vi "Main.vi"() -> ()   [LabVIEW 2015]
uses:
  XYZStage/XYZStage Configuration.ctl
  Camera/Acquisition Settings.ctl
  Automation/ZO Settings.ctl
  Automation/Zstack Settings.ctl
  AOD/AOD Configuration.ctl
  controls/UI Data.ctl
  controls/UI State.ctl
  Settings/Settings.ctl
  Camera/Camera Configuration.ctl
  Logging/Logging Configuration.ctl
  DM/DM Configuration.ctl
  Automation/Automation Configuration.ctl
  V7001/V7001 Configuration.ctl
  <vilib>/vision/Image Controls.llb/IMAQ Image.ctl
  Camera/Camera State.ctl
  Camera/Camera Loop State.ctl
  <vilib>/Utility/miscctls.llb/LVMinMaxIncTypeDef.ctl
  Camera/Live View State.ctl
  DM/DM State.ctl
  DM/DM Loop State.ctl
  V7001/V7001 State.ctl
  V7001/V7001 Loop State.ctl
  AOD/AOD State.ctl
  AOD/AOD Loop State.ctl
  XYZStage/XYZStage State.ctl
  XYZStage/XYZStage Loop State.ctl
  <vilib>/Utility/error.llb/Error Cluster From Error Code.vi
  <vilib>/ErrorRing/Error Ring.xnode
  support/User Event - Stop/Copy of User Event - Stop.lvlib
  support/Message Queue/Message Queue.lvlib
  Camera/Camera.lvlib
  Settings/Settings.lvlib
  Logging/Logging.lvlib
  XYZStage/XYZStage.lvlib
  DM/DM.lvlib
  Automation/Automation.lvlib
  <vilib>/vision/NI_Vision_Development_Module.lvlib
  V7001/V7001.lvlib
  AOD/AOD.lvlib
panel:
  out "Camera Status":bool
  in  "Connect Camera":bool
  in  "X,Y":dbl[](array[slide])=[0.0, 0.0, 0.0, 0.0, 0.0, -0.06565656565656566, 0.0, 0.0, 0.043434343434343436, 0.0, 0.0, 0.0, 0.0, 0.0, 0.0] min=-1.0 max=1.0 scale=-1.0..1.0
  out "AOD Status":string="Disconnected"
  in  "AOD Configuration":T1={"Physical Channel"="Dev1/ao0:1", "Maximum Value"=10.0, "Minimum Value"=1.0, "Update Rate"=192000.0} {"Update Rate" format="%0.2f"; "Minimum Value" format="%0.2f"; "Maximum Value" format="%0.2f"}
  out "AOD Status":bool
  in  "Connect AOD":bool
  in  "Frame":u16(ring)=2 items=["All Off", "All On", "Checkerboard 1", "Random"]
  in  "Test Frame":bool
  out "V7001 Status":string="Disconnected"
  out "V7001 Status":bool
  in  "Connect DMD":bool
  out "XYZ notification":dbl[](array[numeric])
  in  "Move To":bool
  in  "Position in Microns 2":dbl[](array[numeric])
  out "Position in Microns":dbl[](array[numeric])
  in  "Tab Control 2":enum32{"Zernike", "Zstack"}(tab)=enum."Zstack"
  in  "Project and record":bool
  in  "ZO Settings":T2={"Acquisition Settings"={"Save?"=TRUE, "DCIMG Path"=path "E:/test2", "Filename"="beads", "Total Frames"=0, "Sender"=enum."UI"}, "Shift Amplitude"=0.1, "Initial Zernike Vector"=[0.0, 0.0, 0.0, 0.0, 0.0, 0.0, 0.0, 0.0, 0.0, 0.0, 0.0, 0.0, 0.0, 0.0, 0.0]}
  in  "Take Z Stack":bool
  in  "Stop at Current Pos":bool
  in  "Start at Current Pos":bool
  in  "Zstack Settings":T4={"Acquisition Settings"={"Save?"=TRUE, "DCIMG Path"=path "E:/test3", "Filename"="zstacktest1", "Total Frames"=10, "Sender"=enum."UI"}, "XYZ start"=[100.0, 100.0, 100.0], "XYZ end"=[100.0, 100.0, 8282.6875]}
  in  "Stage Stop":bool
  in  "step.size.xy":u16(ring)=6 items=["  1"=1, "  2"=2, "  5"=5, " 10"=10, " 20"=20, " 50"=50, "100"=100]
  in  "Y UP":bool
  in  "X LEFT":bool
  in  "Y DOWN":bool
  in  "X RIGHT":bool
  in  "step.size.z":u16(ring)=6 items=["  1"=1, "  2"=2, "  5"=5, " 10"=10, " 20"=20, " 50"=50, "100"=100]
  in  "Z UP":bool
  in  "Z DOWN":bool
  out "(Basic Histogram)":T5(graph)
  out "Automation Status":string
  in  "Tab Control":enum32{"Manual Trigger", "Live Mode"}(tab)
  in  "Exposure":dbl
  in  "Acquisition Settings":T3={"Save?"=FALSE, "DCIMG Path"=path "E:/test2", "Filename"="test", "Total Frames"=15, "Sender"=enum."UI"}
  in  "Acquire frames":bool
  in  "snap":bool
  out "Acquired Frames":dbl
  in  "Cancel Sequence":bool
  out "Camera Status 3":string
  in  "Go Live":bool
  out "Display":T6(plugin-control)
  in  "Connect DM":bool
  out "Intensity Graph":dbl[][](graph)=[[0.5, 0.5, 0.5, 0.5159398573354096, 0.5288164557874044, 0.535167056900559, 0.5377202162789856, 0.53921067600134, 0.5423702911567251, 0.5, 0.5, 0.5], [0.5, 0.5, 0.4975915358440764, 0.5151805163221181, 0.5235020295826256, 0.5252975455042929, 0.5232956196912321, 0.5202309942220992, 0.5188355241859969, 0.5218457302341335, 0.5, 0.5], [0.5, 0.47468889730160246, 0.5006284404962225, 0.5145729816339067, 0.5192500555540568, 0.5174011321353665, 0.5117547669819483, 0.505045702172458, 0.5000057927959983, 0.49937155950377754, 0.5058738366201876, 0.5], [0.44177297969755197, 0.4797001888362955, 0.5029062478643276, 0.514117304835424, 0.5160608945889862, 0.511478487003708, 0.5030986376837019, 0.4936560887076236, 0.48588269516457605, 0.48251497770576735, 0.48628377065558953, 0.49991687181031336], [0.44693499496071193, 0.4830402937519164, 0.5044244424324095, 0.5138135890559667, 0.5139352684619899, 0.5075309505291726, 0.49732919086162747, 0.4860647315380101, 0.4764694276474235, 0.4712797998410757, 0.4732266824433588, 0.4850378732505436], [0.4495168789955624, 0.4847109132903577, 0.5051837974744415, 0.5136616796015896, 0.5128720945112036, 0.5055565120819772, 0.4944434879180228, 0.4822677640979963, 0.4717611957110005, 0.46566030340824355, 0.46669592151411743, 0.47759584782489306], [0.4495168789955624, 0.4847109132903577, 0.5051837974744415, 0.5136616796015896, 0.5128720945112036, 0.5055565120819772, 0.4944434879180228, 0.4822677640979963, 0.4717611957110005, 0.46566030340824355, 0.46669592151411743, 0.47759584782489306], [0.44693499496071193, 0.4830402937519164, 0.5044244424324095, 0.5138135890559667, 0.5139352684619899, 0.5075309505291726, 0.49732919086162747, 0.4860647315380101, 0.4764694276474235, 0.4712797998410757, 0.4732266824433588, 0.4850378732505436], [0.44177297969755197, 0.4797001888362955, 0.5029062478643276, 0.514117304835424, 0.5160608945889862, 0.511478487003708, 0.5030986376837019, 0.4936560887076236, 0.48588269516457605, 0.48251497770576735, 0.48628377065558953, 0.49991687181031336], [0.5, 0.47468889730160246, 0.5006284404962225, 0.5145729816339067, 0.5192500555540568, 0.5174011321353665, 0.5117547669819483, 0.505045702172458, 0.5000057927959983, 0.49937155950377754, 0.5058738366201876, 0.5], [0.5, 0.5, 0.4975915358440764, 0.5151805163221181, 0.5235020295826256, 0.5252975455042929, 0.5232956196912321, 0.5202309942220992, 0.5188355241859969, 0.5218457302341336, 0.5, 0.5], [0.5, 0.5, 0.5, 0.5159398573354096, 0.5288164557874044, 0.535167056900559, 0.5377202162789856, 0.53921067600134, 0.5423702911567251, 0.5, 0.5, 0.5]]
  in  "DM Tab Control":enum32{"Setup", "Zernike Modes", "Other"}(tab)=enum."Zernike Modes"
  in  "DM Serial":string="C18W147#040"
  in  "zoom sliders":bool=TRUE
  in  "Sliders to text":bool
  in  "Zero zernike":bool
  in  "Zernike Amplitudes":dbl[](array[slide])=[0.0, 0.0, 0.0, 0.0, 0.0, -0.06565656565656566, 0.0, 0.0, 0.043434343434343436, 0.0, 0.0, 0.0, 0.0, 0.0, 0.0] scale=-0.1..0.1
  in  "Matlab Paste":string
  in  "Set Z from paste":bool
  out "DM Status":bool
  out "DM Status":string="Disconnected"
  in  "XYZ Stage Configuration":T7={"VISA resource name"="COM3", "Timeout (3sec)"=3000}
  out "XYZ Status":string
  out "XYZ Status":bool
  in  "Connect XYZ stage":bool
  in  "Exit":bool
  in  "Stop":bool
  in  "Settings":bool
  out "Status":string="Exit"
  in  "Start":bool
  # "XYZ STAGE"
  # "CAMERA"
  # "abs  pos."
  # "x"
  # "y"
  # "z"
  # "DEFORMABLE MIRROR"
  # "AUTOMATION"
  # "To Do:\n\n'live' camera mode\nbetter image display\nbetter camera settings control\n(especially fov)\nZstack! (in automation loop...)\narrows etc for translation stage UI\ntable of zernike amplitudes (to easily cycle through)\n\n\nDone:\n\nmake 'automation' loop which does this sequence:\nsend zernike to DM\ntrigger camera exposure\nanalyze camera data\ncalculates optimal DM configuration\n\nadd data stream so UI can display most recent 'Live' camera frame."
  # "DMD"
  # "-Connect/disconnect\n-Static:\n--Apply mask in DMD coordinates\n--Apply mask in Camera coordinates\n--Configure DMD<->Camera mapping\n-Dynamic:\n--upload sequence and trigger settings\n--play sequence...\n--sequence play settings..."
  # "AOD"
  # "Put Camera into software triggered sequence mode."
  # "To Do:\nAdd these settings:\n-exposure time\n-Frame rate\n-Binning\n-subregion\nDisplay Current Frame Rate\nUpdate camera Status..."
  # "Piston"
  # "Tilt X"
  # "Tilt Y"
  # "Ast H"
  # "Defocus"
  # "Ast D"
  # "3rd Spherical"
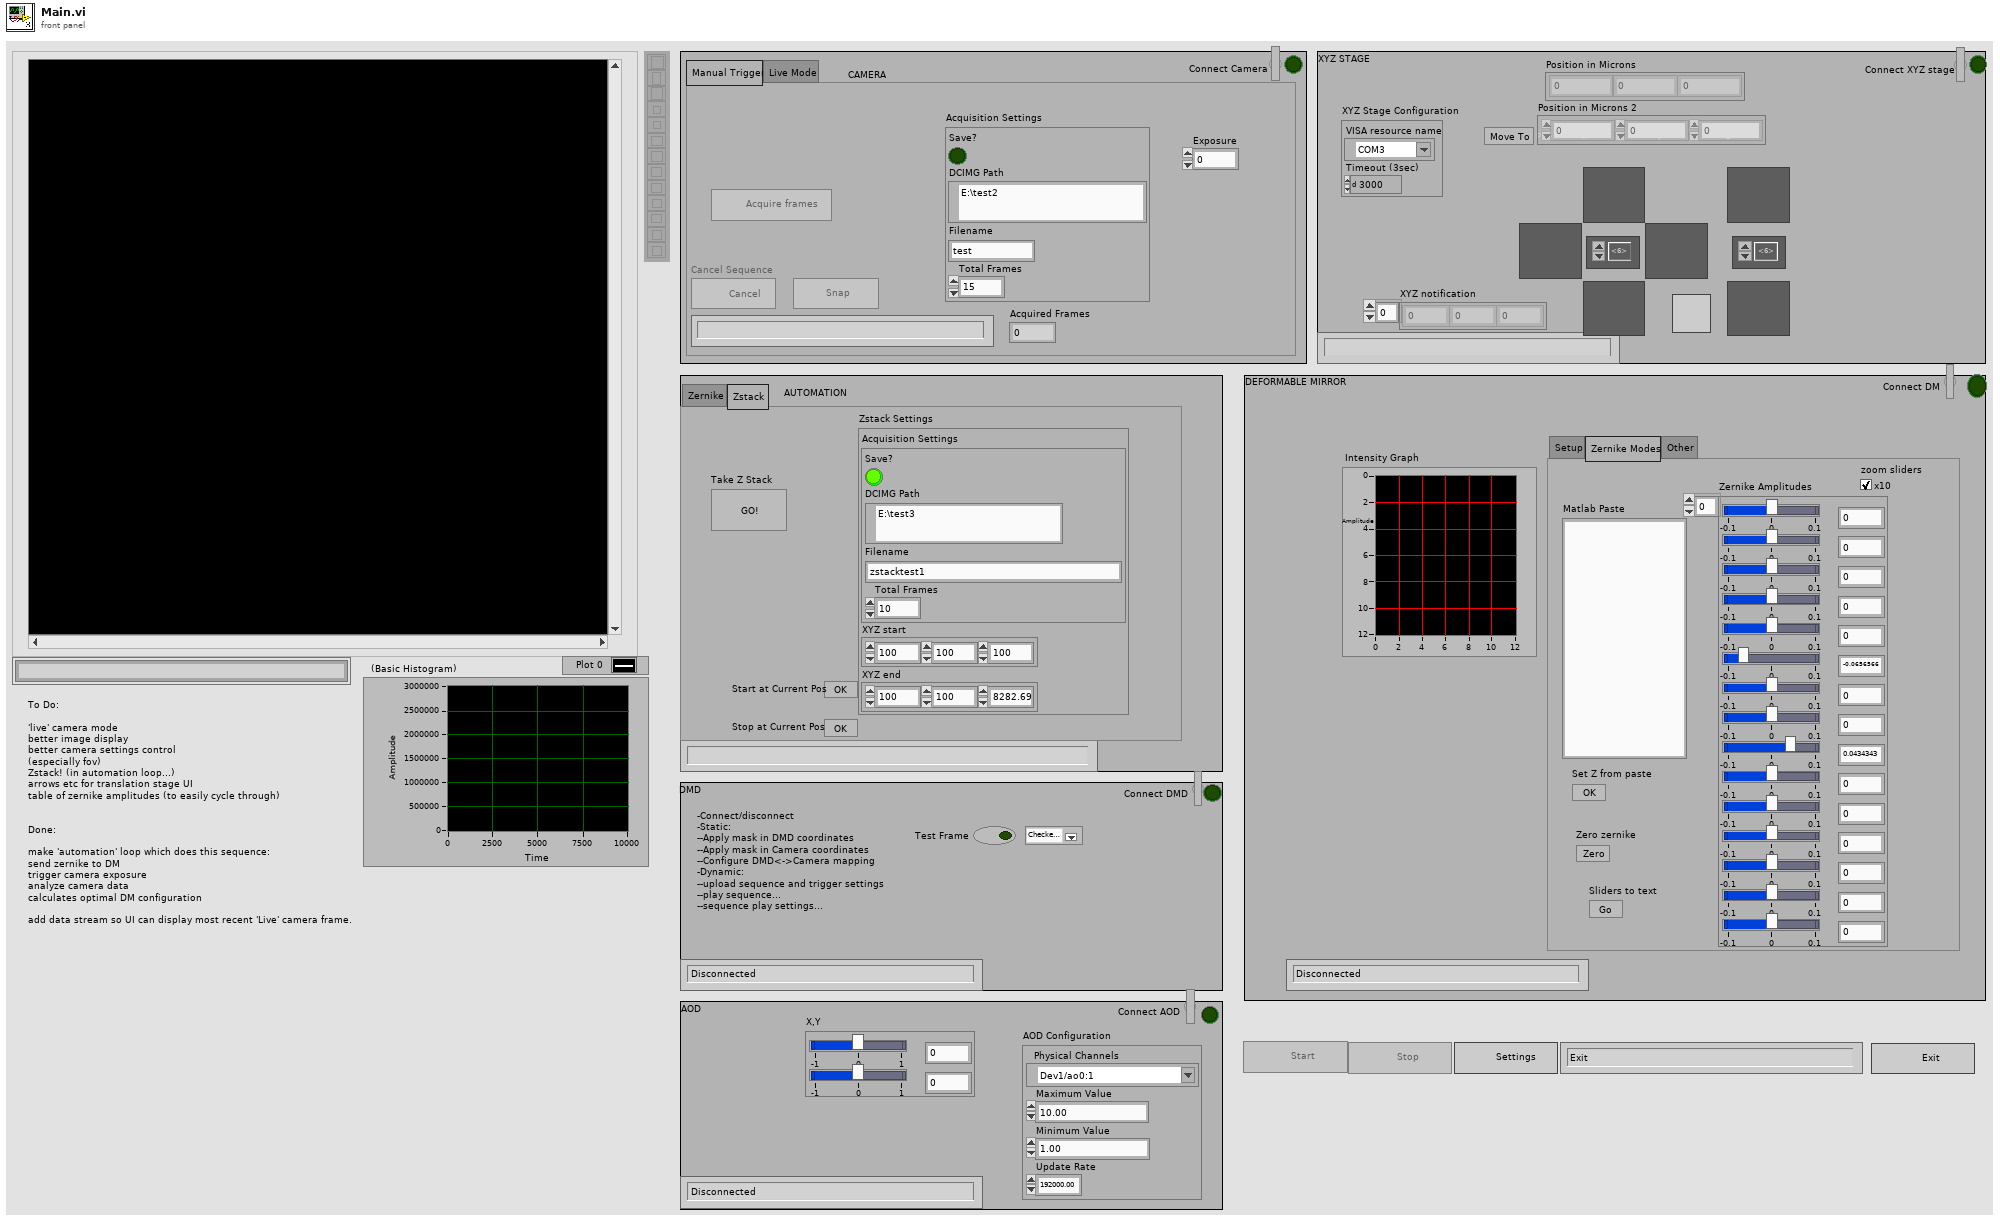
[diagram p1: front panel]
types:
  T1 = typedef "AOD.lvlib/AOD Configuration.ctl" = cluster{"Physical Channel":tag, "Maximum Value":dbl, "Minimum Value":dbl, "Update Rate":dbl}
  T2 = typedef "Automation.lvlib/ZO Settings.ctl" = cluster{"Acquisition Settings":T3, "Shift Amplitude":dbl, "Initial Zernike Vector":dbl[]}
  T3 = typedef "Camera.lvlib/Acquisition Settings.ctl" = cluster{"Save?":bool, "DCIMG Path":path, "Filename":string, "Total Frames":i32, "Sender":enum16{"UI", "Automation"}}
  T4 = typedef "Automation.lvlib/Zstack Settings.ctl" = cluster{"Acquisition Settings":T3, "XYZ start":dbl[], "XYZ end":dbl[]}
  T5 = cluster{"Starting Value":sgl, "Incremental Value":sgl, "Histogram":u32[]}
  T6 = typedef "IMAQ Image.ctl" = refnum<image>
  T7 = typedef "XYZStage.lvlib/XYZStage Configuration.ctl" = cluster{"VISA resource name":refnum<visa-resource-name>, "Timeout (3sec)":u32}
  T8 = typedef "Settings.lvlib/Settings.ctl" = cluster{"Camera Configuration":T9, "Logging Configuration":T10, "XYZ Configuration":T7, "DM Configuration":T11, "Automation Configuration":T12, "V7001 Configuration":T13, "AOD Configuration":T1}
  T9 = typedef "Camera.lvlib/Camera Configuration.ctl" = cluster{"Camera Index":u32}
  T10 = typedef "Logging.lvlib/Logging Configuration.ctl" = cluster{"Log File Base Path":path}
  T11 = typedef "DM.lvlib/DM Configuration.ctl" = cluster{"Selected Profile":string, "dm out":cluster{"type":i32, "ID":i32, "size":i32, "@dummy control@":i8, "@dummy control@":i8, "@dummy control@":i8, "@dummy control@":i8, "lutName":u64}}
  T12 = typedef "Automation.lvlib/Automation Configuration.ctl" = cluster{" Index":u32}
  T13 = typedef "V7001.lvlib/V7001 Configuration.ctl" = cluster{" Index":u32}
  T14 = typedef "UI State.ctl" = enum16{"Idle", "ZStack"}
  T15 = typedef "UI Data.ctl" = cluster{"Start Ref":refnum<vi>, "Stop Ref":refnum<vi>, "Settings Ref":refnum<vi>, "Exit Ref":refnum<vi>, "Status Ref":refnum<vi>, "Data Ref":refnum<vi>, "Camera Status Light Ref":refnum<vi>, "Camera Switch":refnum<vi>, "Acquire frames ref":refnum<vi>, "snap button ref":refnum<vi>, "XYZ Switch":refnum<vi>, "XYZ Status Light Ref":refnum<vi>, "Move button ref":refnum<vi>, "DM Switch ref":refnum<vi>, "DM Status Light Ref":refnum<vi>, "Zernike Amplitudes":refnum<vi>, "Position in Microns":refnum<vi>, "V7001 Status Light Ref":refnum<vi>, "V7001 Switch Ref":refnum<vi>, "AOD Status Light Ref":refnum<vi>, "AOD Switch Ref":refnum<vi>}
  T16 = typedef "Message Queue.lvlib/All Message Queues.ctl" = cluster{"UI":refnum<queue>, "XYZStage":refnum<queue>, "Camera":refnum<queue>, "DM":refnum<queue>, "Automation":refnum<queue>, "V7001":refnum<queue>, "AOD":refnum<queue>}
  T17 = typedef "Camera.lvlib/Camera State.ctl" = cluster{"Camera State":T18, "Current Frame":i32, "Handle out":u32, "Camera Details":cluster{"Model":string, "Camera ID":string, "Firmware":string}, "Sub Region":cluster{"H Offset":cluster{"Value":i32, "Limits":T19}, "V Offset":cluster{"Value":i32, "Limits":T19}, "H Size":cluster{"Value":i32, "Limits":T19}, "V Size":cluster{"Value":i32, "Limits":T19}}, "Acquisition Settings":T3, "Live View State":T20}
  T18 = typedef "Camera.lvlib/Camera Loop State.ctl" = enum16{"Idle", "Live View", "Ready", "Acquiring"}
  T19 = typedef "LVMinMaxIncTypeDef.ctl" = cluster{"Minimum":dbl, "Maximum":dbl, "Increment":dbl}
  T20 = typedef "Camera.lvlib/Live View State.ctl" = cluster{"Loop Counter":i32, "Time Of Latest Frame":u32, "Frame Count":u32, "FPS frames":dbl, "FPS Time":u32, "Current FPS":dbl}
  T21 = enum8{"Enabled", "Disabled", "Disabled and Grayed Out"}
  T22 = typedef "DM.lvlib/DM State.ctl" = cluster{"DM State":T23, "Last Image Sent":dbl[][], "Flatmap":dbl[], "Flatmap Path":path, "Matlab Directory Path":path}
  T23 = typedef "DM.lvlib/DM Loop State.ctl" = enum16{"Idle", "Connected"}
  T24 = typedef "V7001.lvlib/V7001 State.ctl" = cluster{"V7001 State":T25, "Handle out":u32, "Size":dbl[]}
  T25 = typedef "V7001.lvlib/V7001 Loop State.ctl" = enum16{"Idle", "Connected"}
  T26 = typedef "AOD.lvlib/AOD State.ctl" = cluster{"AOD State":T27, "daq task":refnum<k21>, "AOD Configuration":T1}
  T27 = typedef "AOD.lvlib/AOD Loop State.ctl" = enum16{"Idle", "Connected"}
  T28 = typedef "XYZStage.lvlib/XYZStage State.ctl" = cluster{"XYZStage State":T29, "Handle out":u32, "VISA resource name":refnum<visa-resource-name>, "num controllers connected":u8, "Connector statuses":u8[], "Position in Microns":dbl[], "measured manipulator":u8}
  T29 = typedef "XYZStage.lvlib/XYZStage Loop State.ctl" = enum16{"Idle", "Connected", "Moving"}
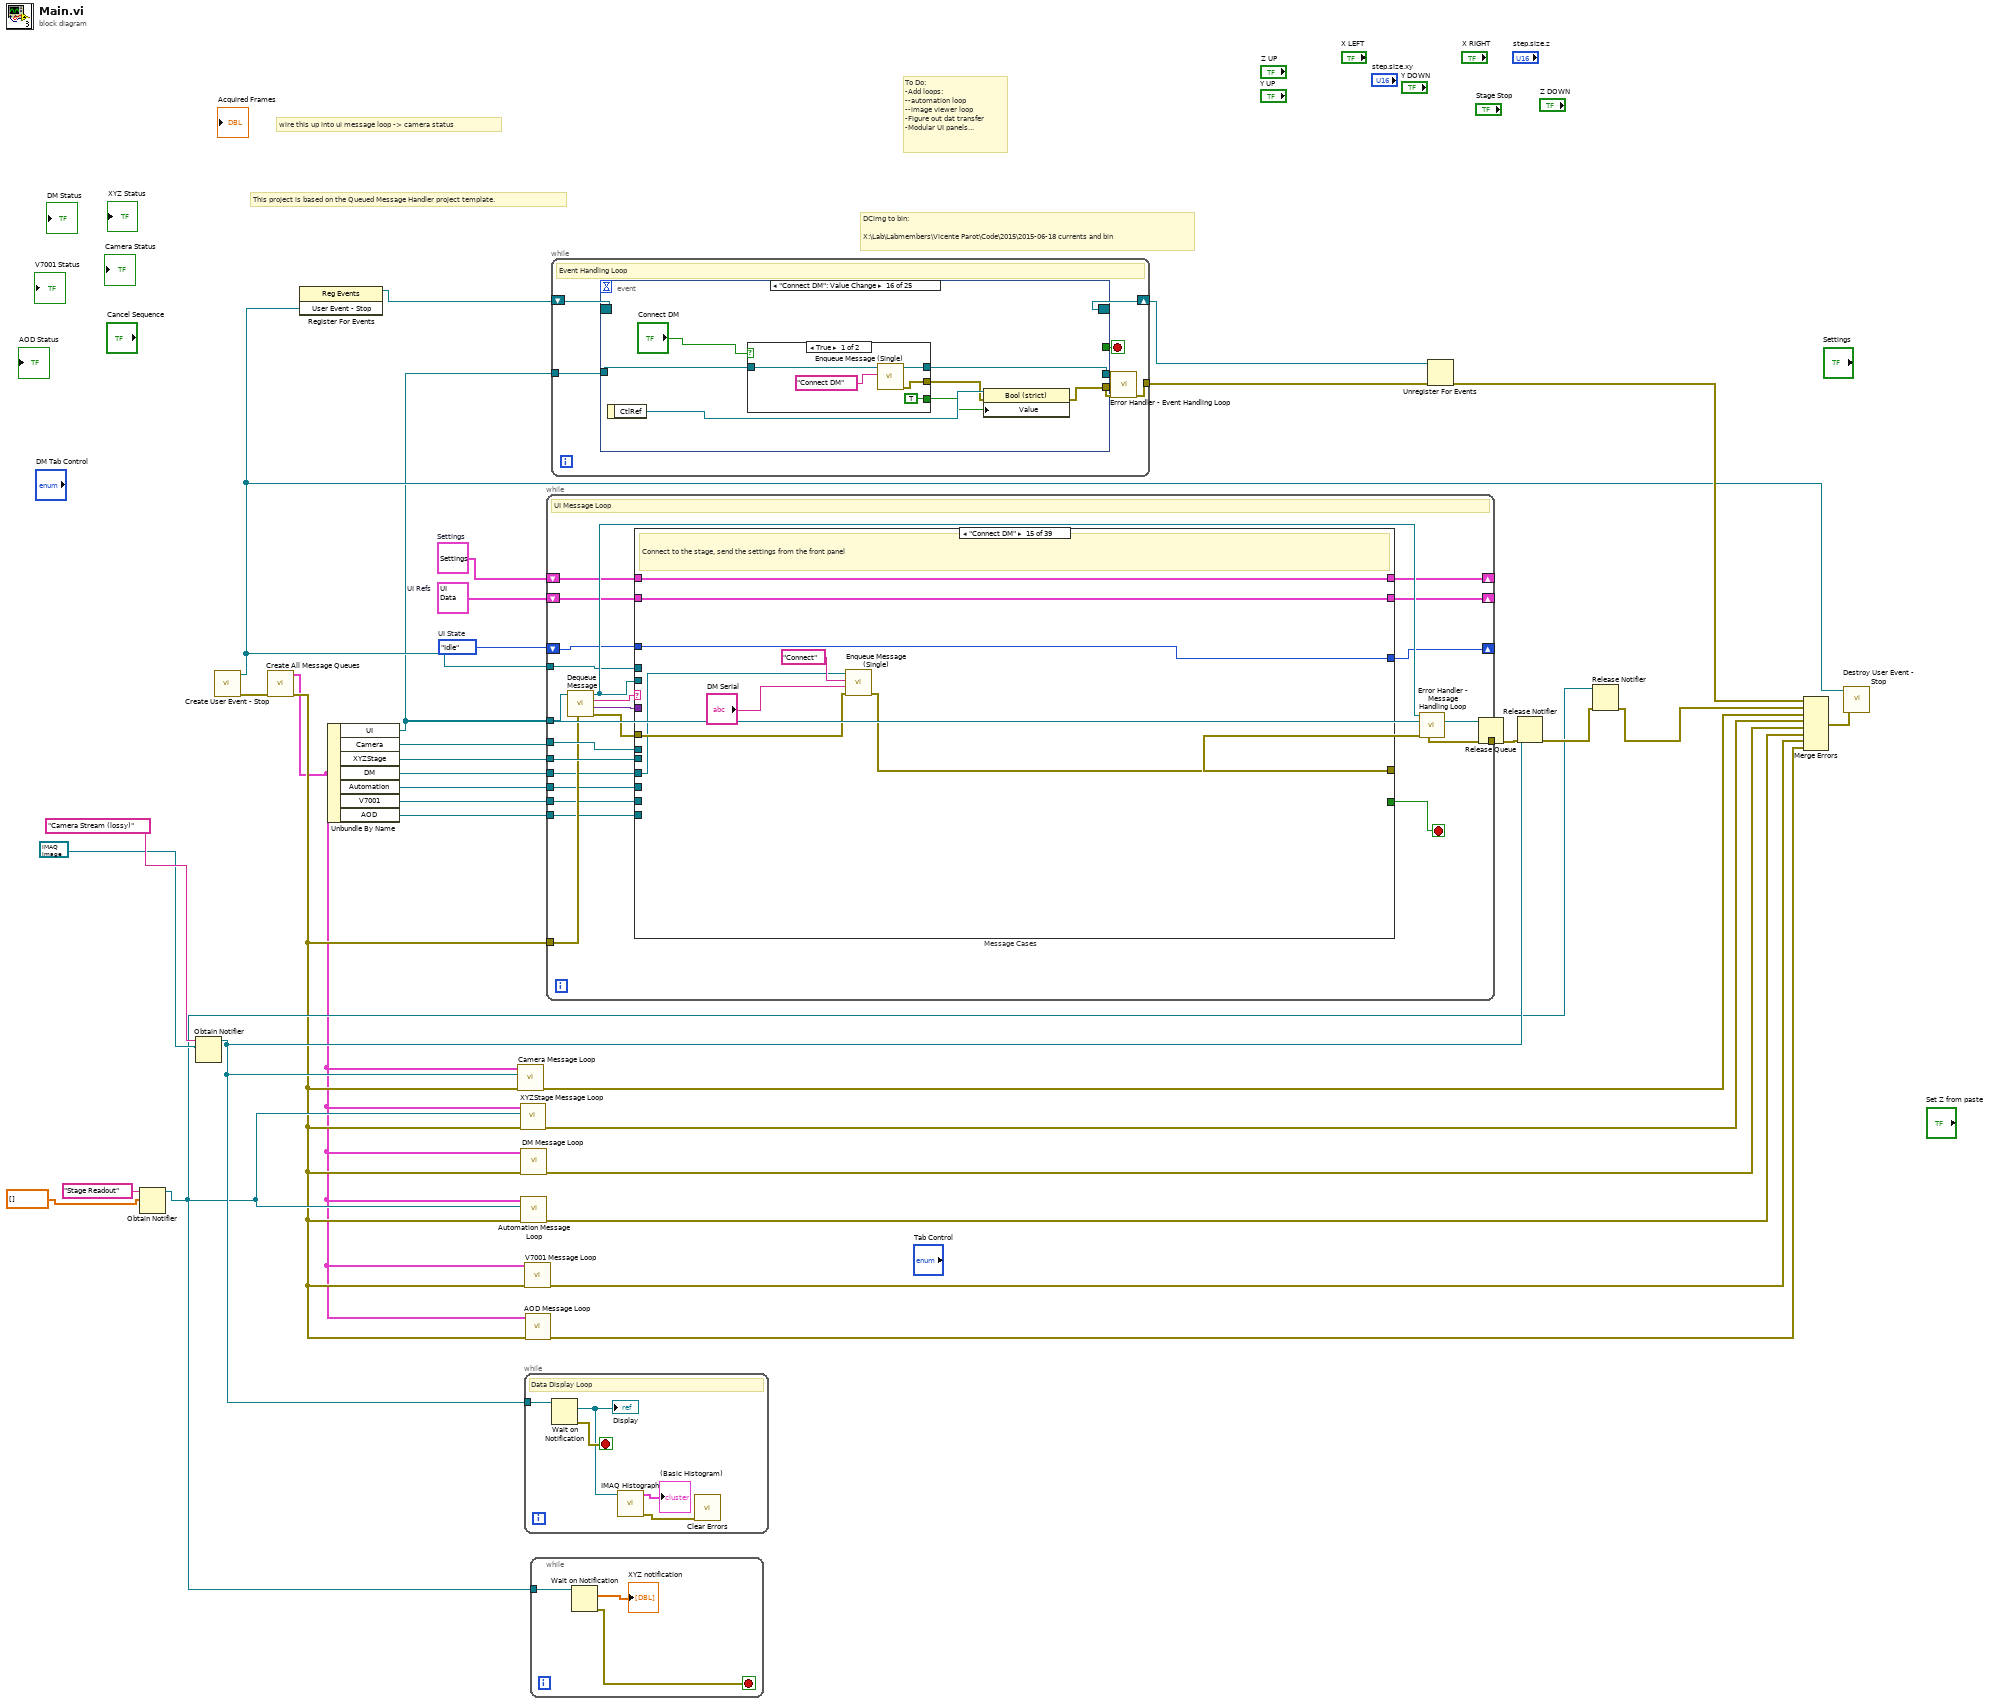
[diagram p0: block diagram]
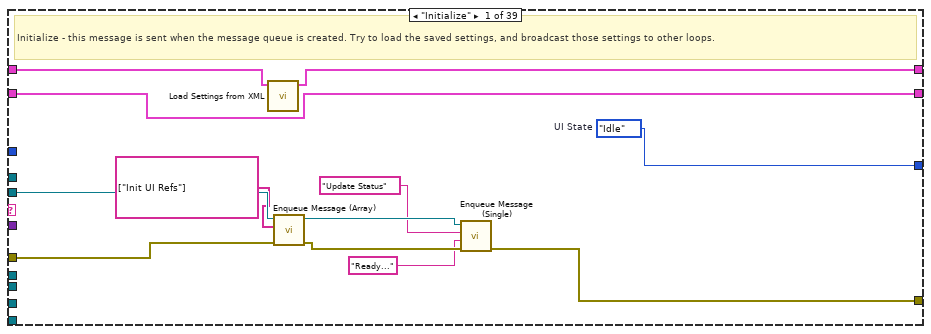
[diagram p2: hidden frame]
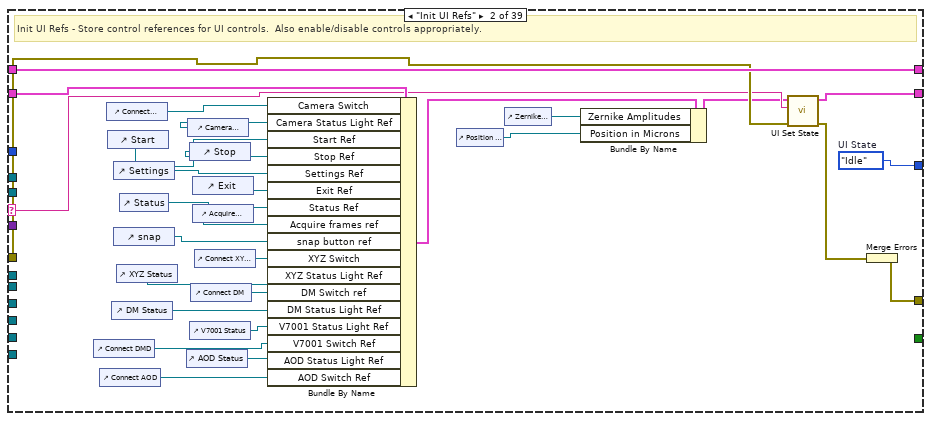
[diagram p3: hidden frame]
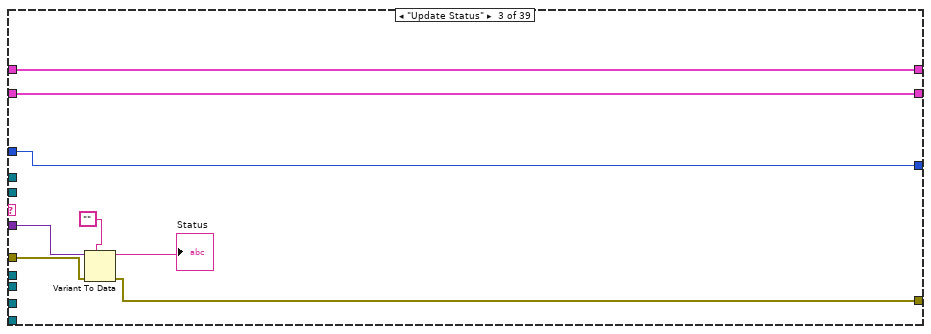
[diagram p4: hidden frame]
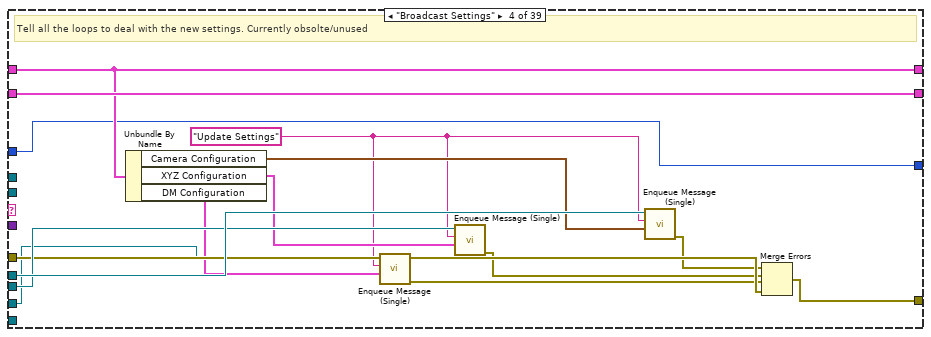
[diagram p5: hidden frame]
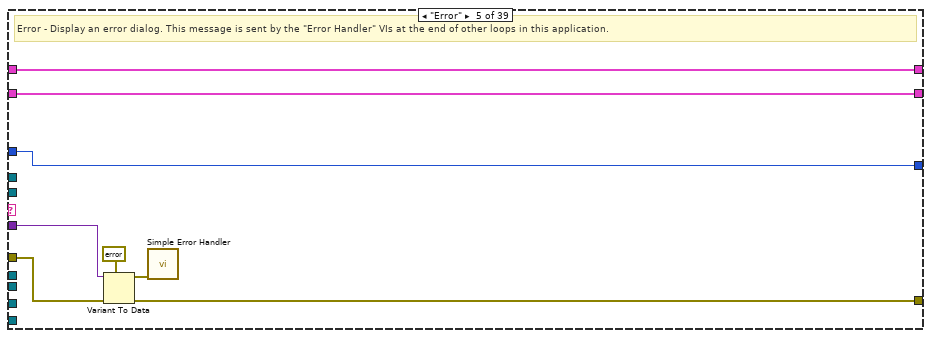
[diagram p6: hidden frame]
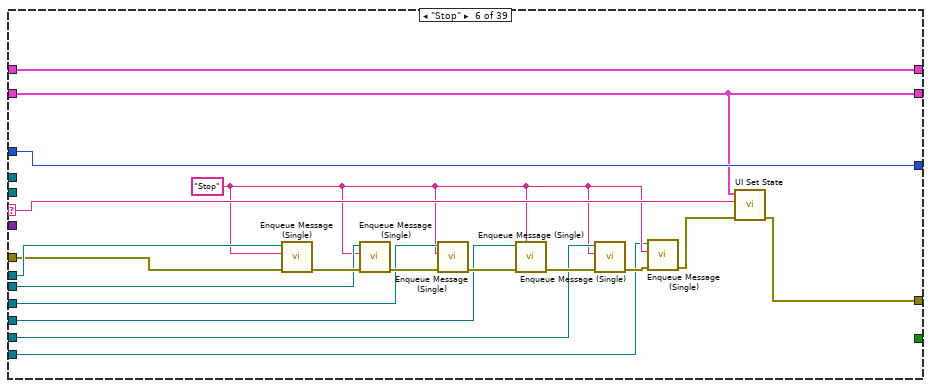
[diagram p7: hidden frame]
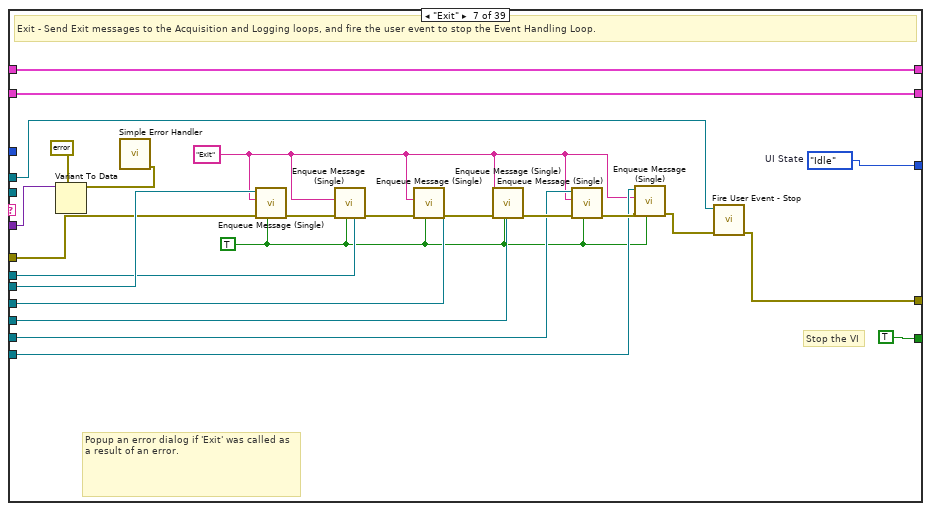
[diagram p8: hidden frame]
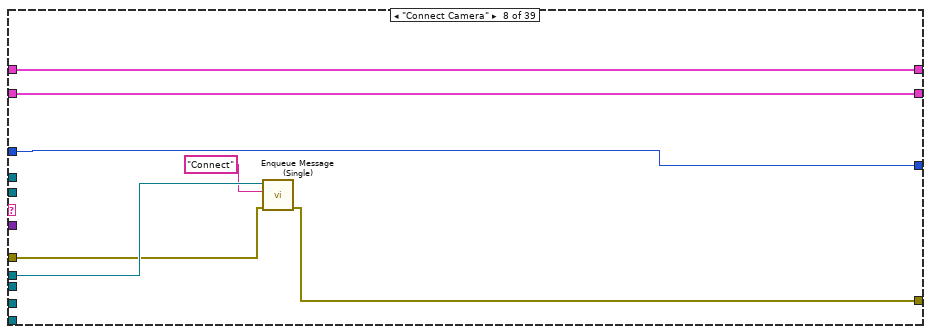
[diagram p9: hidden frame]
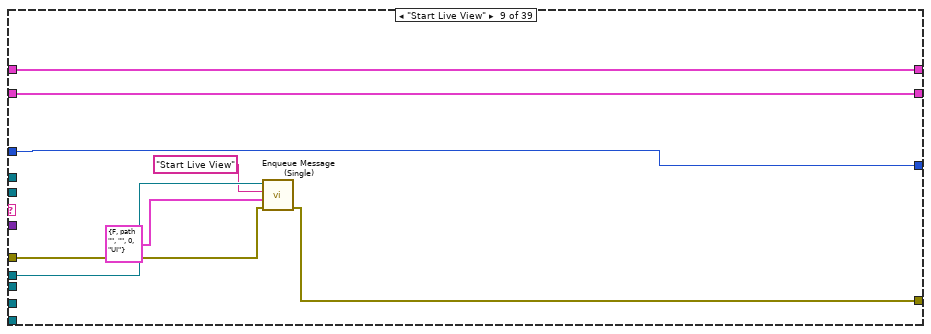
[diagram p10: hidden frame]
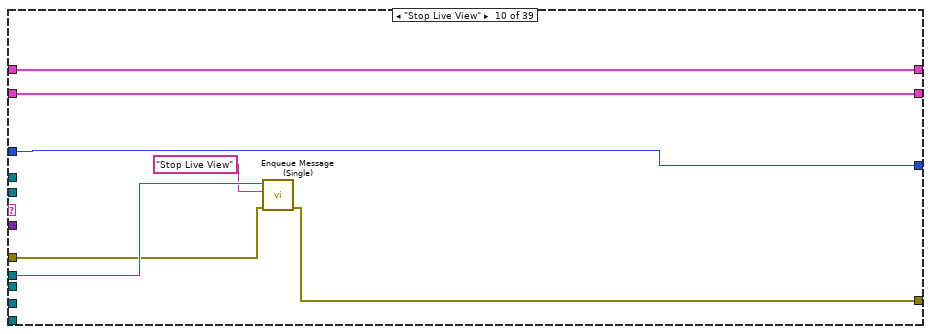
[diagram p11: hidden frame]
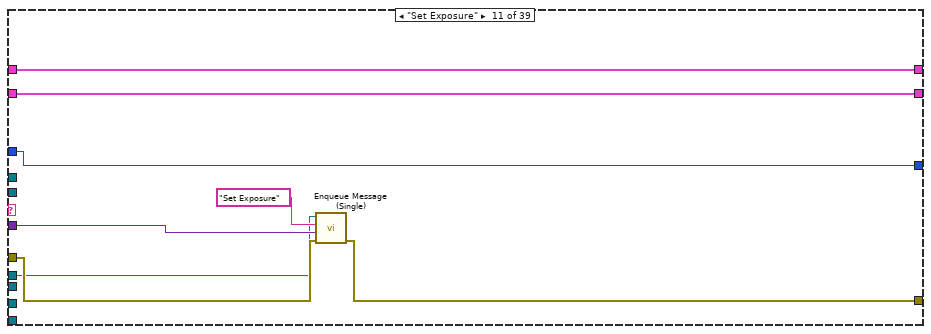
[diagram p12: hidden frame]
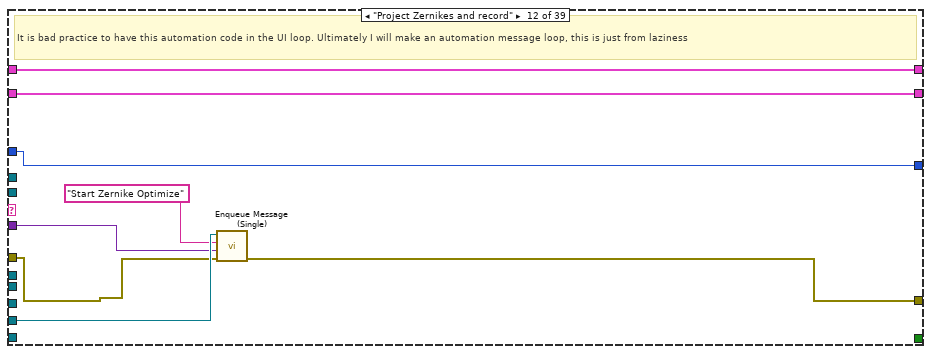
[diagram p13: hidden frame]
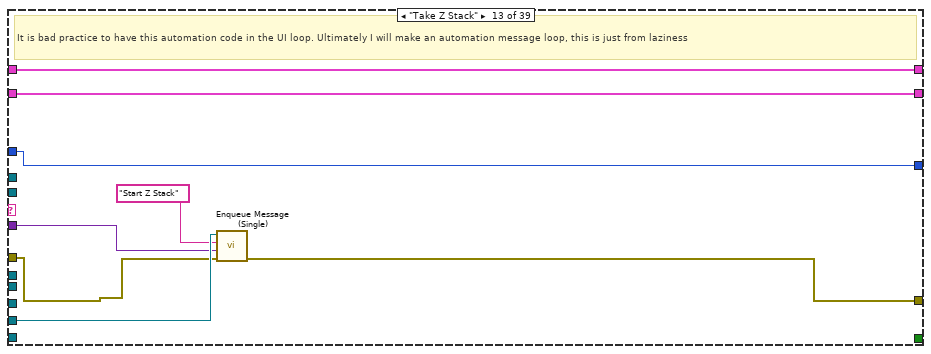
[diagram p14: hidden frame]
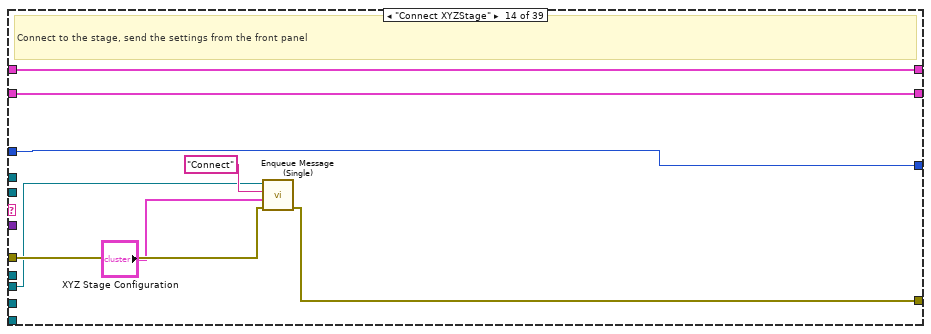
[diagram p15: hidden frame]
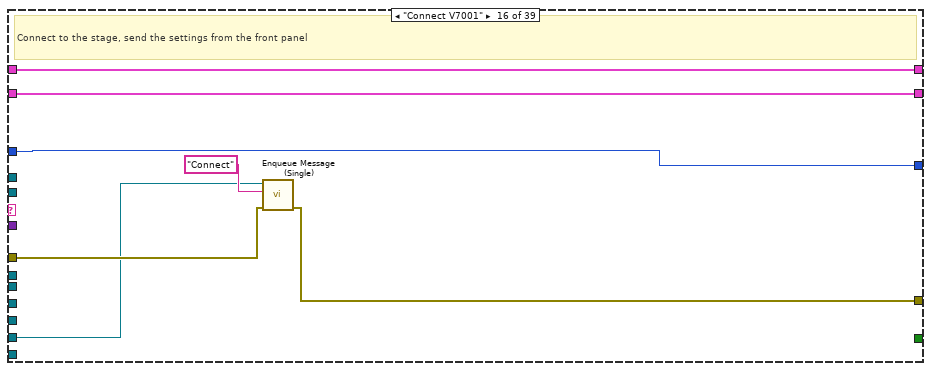
[diagram p16: hidden frame]
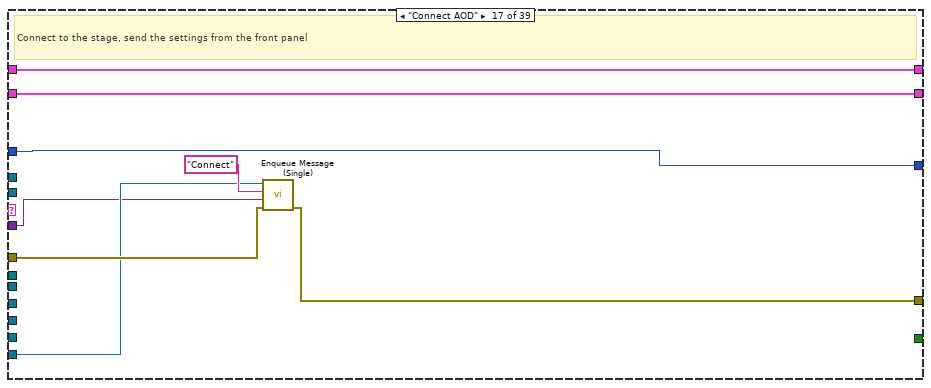
[diagram p17: hidden frame]
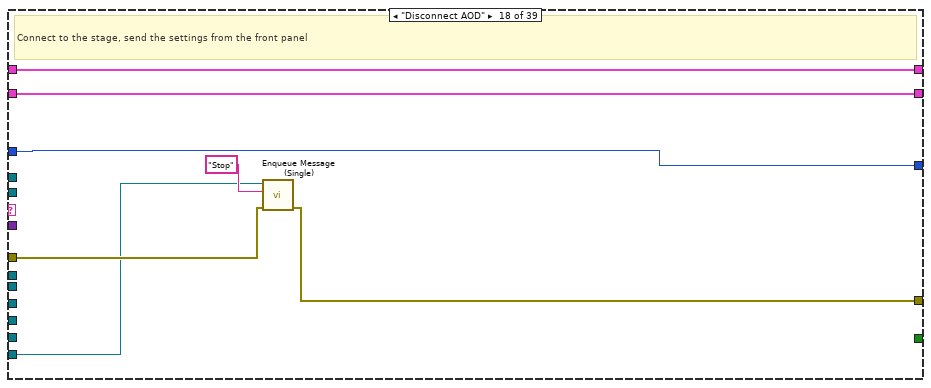
[diagram p18: hidden frame]
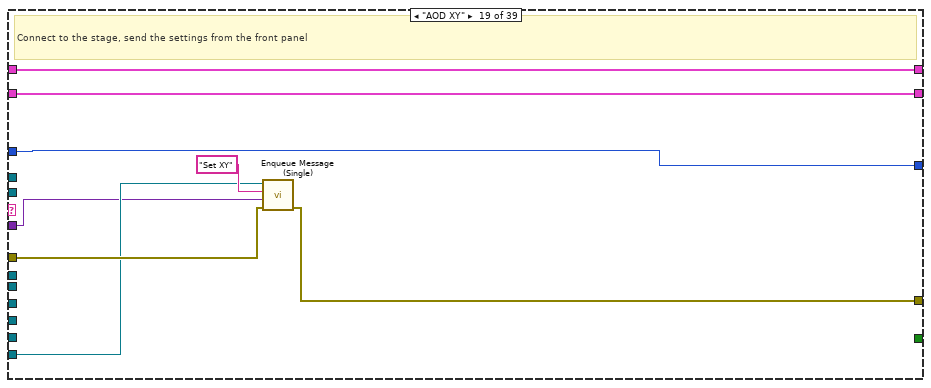
[diagram p19: hidden frame]
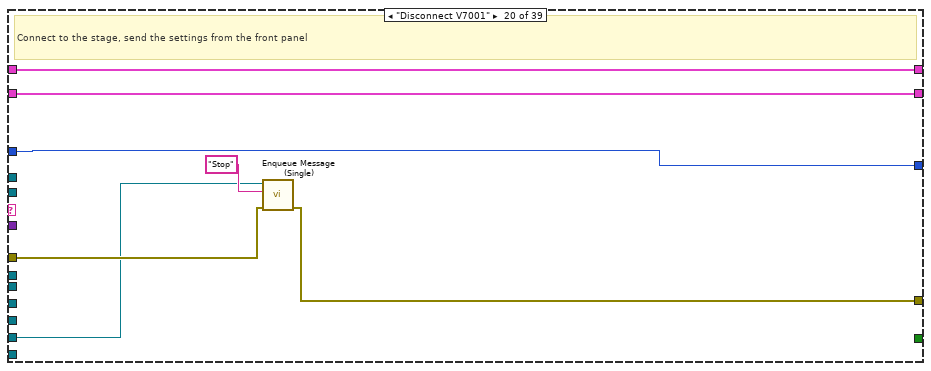
[diagram p20: hidden frame]
diagram:
  w23 = T8 {"Camera Configuration"={"Camera Index"=0}, "Logging Configuration"={"Log File Base Path"=path ""}, "XYZ Configuration"={"VISA resource name"="", "Timeout (3sec)"=0}, "DM Configuration"={"Selected Profile"="", "dm out"={"type"=0, "ID"=0, "size"=0, "@dummy control@"=0, "@dummy control@"=0, "@dummy control@"=0, "@dummy control@"=0, "lutName"=0}}, "Automation Configuration"={" Index"=0}, "V7001 Configuration"={" Index"=0}, "AOD Configuration"={"Physical Channel"="Dev1/ao0:1", "Maximum Value"=0.0, "Minimum Value"=1.0, "Update Rate"=192000.0}}  # Settings
  w28 = UI_State."Idle"  # UI State
  w27 = T15 {"Start Ref"=refnum, "Stop Ref"=refnum, "Settings Ref"=refnum, "Exit Ref"=refnum, "Status Ref"=refnum, "Data Ref"=refnum, "Camera Status Light Ref"=refnum, "Camera Switch"=refnum, "Acquire frames ref"=refnum, "snap button ref"=refnum, "XYZ Switch"=refnum, "XYZ Status Light Ref"=refnum, "Move button ref"=refnum, "DM Switch ref"=refnum, "DM Status Light Ref"=refnum, "Zernike Amplitudes"=refnum, "Position in Microns"=refnum, "V7001 Status Light Ref"=refnum, "V7001 Switch Ref"=refnum, "AOD Status Light Ref"=refnum, "AOD Switch Ref"=refnum}  # UI Refs
  # "DCimg to bin:\n\nX:\\Lab\\Labmembers\\Vicente Parot\\Code\\2015\\2015-06-18 currents and bin"
  # "To Do:\n-Add loops:\n--automation loop\n--image viewer loop\n-Figure out dat transfer\n-Modular UI panels..."
  # "wire this up into ui message loop -> camera status"
  # "This project is based on the Queued Message Handler project template."
  n1 = Obtain Notifier(name (unnamed)="Stage Readout", notification data type=dbl[] [] ("Position in Microns")) -> (notifier out=w8:refnum<notifier>)  [unwired: 2 in, 2 out]
  n2 = Obtain Notifier(name (unnamed)="Camera Stream (lossy)", notification data type=T6 refnum ("New Image")) -> (notifier out=w13:refnum<notifier>)  [unwired: 2 in, 2 out]
  n3 = call "Create User Event - Stop.vi"() -> ("error out"=w33:errorcluster, "User Event - Stop"=w24:refnum<user-event>)  [unwired: 10 in]
  n4 = call "Create All Message Queues.vi"("error in (no error)"=w33) -> ("error out"=w4:errorcluster, "Message Queues out"=w3:T16)  [unwired: 9 in]
  n5 = register-events(w24) -> (reference out=w35:refnum<event-registration>)  [unwired: 2 in, 1 out]
  n6 = Unbundle By Name(w3) -> ("UI"=w6:refnum<queue>, "Camera"=w25:refnum<queue>, "XYZStage"=w26:refnum<queue>, "DM"=w19:refnum<queue>, "Automation"=w14:refnum<queue>, "V7001"=w5:refnum<queue>, "AOD"=w1:refnum<queue>)
  n7 = call "Camera Message Loop.vi"("error in (no error)"=w4, "Data Notifier"=w13, "Message Queues"=w3) -> ("error out"=w22:errorcluster)  [unwired: 8 in]
  n8 = call "XYZStage Message Loop.vi"("error in (no error)"=w4, "Stage Readout Notifier"=w8, "Message Queues"=w3) -> ("error out"=w21:errorcluster)  [unwired: 8 in]
  n9 = call "DM Message Loop.vi"("error in (no error)"=w4, "Message Queues"=w3) -> ("error out"=w20:errorcluster)  [unwired: 9 in]
  n10 = call "Automation Message Loop.vi"("error in (no error)"=w4, "Stage Readout Notifier"=w8, "Message Queues"=w3) -> ("error out"=w15:errorcluster)  [unwired: 8 in]
  n11 = call "V7001 Message Loop.vi"("error in (no error)"=w4, "Message Queues"=w3) -> ("error out"=w7:errorcluster)  [unwired: 9 in]
  n12 = while "Data Display Loop" {
    tunnel: w13 -> [w40]
    stop <- w39 stop-if-true
    # "Data Display Loop"
    n13 = Wait on Notification(notifier=w40) -> (notification=w38:T6, error out=w39:errorcluster)  [unwired: 3 in, 2 out]
    "Display" <- w38
    n14 = call "IMAQ Histograph"("Image"=w38) -> ("error out"=w36:errorcluster, "Histogram Graph"=→"(Basic Histogram)":T5)  [unwired: 7 in, 2 out]
    n15 = call <vilib>:"Clear Errors.vi"("error in (no error)"=w36) -> ()  [unwired: 5 in, 2 out]
  }
  n16 = call "AOD Message Loop.vi"("error in (no error)"=w4, "Message Queues"=w3) -> ("error out"=w2:errorcluster)  [unwired: 9 in]
  n17 = while {
    tunnel: w8 -> [w42]
    stop <- w43 stop-if-true
    n18 = Wait on Notification(notifier=w42) -> (notification=→"XYZ notification":dbl[], error out=w43:errorcluster)  [unwired: 3 in, 2 out]
  }
  n19 = while {
    tunnel: w6 -> [w65]
    tunnel: [w61] -> w29
    shift-right: [w58] -> _
    shift-left: w28 -> [w59]
    shift-right: [w56] -> _
    shift-left: w27 -> [w57]
    tunnel: w26 -> [w54]
    tunnel: w25 -> [w53]
    tunnel: w24 -> [w52]
    shift-right: [w49] -> _
    shift-left: w23 -> [w50]
    tunnel: w4 -> [w48]
    tunnel: w19 -> [w47]
    tunnel: w14 -> [w46]
    tunnel: w5 -> [w45]
    tunnel: w1 -> [w44]
    stop <- w51 stop-if-true
    # "UI Message Loop"
    n20 = call "Dequeue Message.vi"("error in (no error)"=w48, "Message Queue"=w65) -> ("error out"=w63:errorcluster, "Message Data"=w55:variant, "Message"=w64:string, "dup Message Queue"=w60:refnum<queue>)  [unwired: 6 in]
    n21 = case "Message Cases" shown="\"Connect DM\"" w64 {
      selector: w64 -> [_ w94 _ _ _ w154 _ _ _ _ _ _ _ _ _ _ _ _ _ _ _ _ _ _ _ _ _ _ _ _ _ _ _ _ _ _ _ _ w508]
      tunnel: w60 -> [w77 _ _ _ _ _ _ _ _ _ _ _ _ _ _ _ _ _ _ _ _ _ _ _ _ _ _ _ _ _ _ _ _ _ _ _ _ _ _]
      tunnel: w63 -> [w75 w95 w111 w123 w134 w150 w176 w183 w191 w198 w206 w215 w223 w231 w239 w246 w254 w261 w269 w276 w282 w291 w299 w304 w326 w343 w352 w359 w367 w373 w381 w389 w402 w435 w453 w470 w487 w505 _]
      tunnel: [w70 w97 w110 w124 w132 w152 w173 w182 w190 w197 w205 w214 w222 w230 w238 w245 w253 w260 w268 w275 w281 w290 w298 w303 w314 w345 w351 w358 w366 w372 w380 w388 w402 w435 w453 w470 w487 w505 w507] -> w62
      tunnel: w59 -> [_ _ w109 w121 w131 w156 _ w181 w189 w196 w210 w211 w219 w229 w237 w244 w252 w259 w267 w274 w287 w289 w297 w313 w332 w347 w350 w357 w365 w371 w379 w387 w397 w430 w448 w465 w482 w501 w506]
      tunnel: [w69 w102 w109 w121 w131 w156 w179 w181 w189 w196 w210 w211 w219 w229 w237 w244 w252 w259 w267 w274 w287 w289 w297 w313 w332 w347 w350 w357 w365 w371 w379 w387 w397 w430 w448 w465 w482 w501 w506] -> w58
      tunnel: w57 -> [w68 w101 w108 w129 w137 w153 w180 w187 w195 w202 w209 w218 w226 w234 w242 w249 w257 w264 w272 w279 w286 w294 w302 w308 w329 w346 w355 w362 w370 w377 w385 w393 w398 w431 w449 w466 w483 w502 w510]
      tunnel: [w68 w91 w108 w129 w137 w153 w180 w187 w195 w202 w209 w218 w226 w234 w242 w249 w257 w264 w272 w279 w286 w294 w302 w308 w329 w346 w355 w362 w370 w377 w385 w393 w398 w431 w449 w466 w483 w502 w510] -> w56
      tunnel: w55 -> [_ _ w112 _ w133 _ w170 _ _ _ w204 w213 w221 _ _ _ w250 _ w265 _ w280 _ w295 w311 w330 w344 _ _ w363 _ w378 w386 w400 w433 w451 w468 w485 w503 _]
      tunnel: w54 -> [_ _ _ w126 _ w148 w178 _ _ _ _ _ _ w228 _ _ _ _ _ _ _ _ _ _ _ _ w349 w356 w364 _ _ _ _ _ _ _ _ _ _]
      tunnel: w53 -> [_ _ _ w128 _ w151 w177 w185 w193 w200 w203 _ _ _ _ _ _ _ _ _ _ _ _ _ _ _ _ _ _ w375 w383 w391 _ _ _ _ _ _ _]
      tunnel: w52 -> [_ _ _ _ _ _ w174 _ _ _ _ _ _ _ _ _ _ _ _ _ _ _ _ _ _ _ _ _ _ _ _ _ _ _ _ _ _ _ _]
      tunnel: [_ _ _ _ _ _ TRUE _ _ _ _ _ _ _ _ _ _ _ _ _ _ _ _ _ _ _ _ _ _ _ _ _ _ _ _ _ _ _ _] -> w51
      tunnel: w50 -> [w66 w99 w107 w122 w130 w155 w171 w186 w194 w201 w208 w217 w225 w233 w241 w248 w256 w263 w271 w278 w285 w293 w301 w312 w331 w348 w354 w361 w369 w376 w384 w392 w401 w434 w452 w469 w486 w504 w509]
      tunnel: [w67 w99 w107 w122 w130 w155 w171 w186 w194 w201 w208 w217 w225 w233 w241 w248 w256 w263 w271 w278 w285 w293 w301 w312 w331 w348 w354 w361 w369 w376 w384 w392 w401 w434 w452 w469 w486 w504 w509] -> w49
      tunnel: w47 -> [_ _ _ w116 _ w146 w166 _ _ _ _ _ _ _ w236 _ _ _ _ _ _ w288 w296 _ _ _ _ _ _ _ _ _ _ _ _ _ _ _ _]
      tunnel: w46 -> [_ _ _ _ _ w144 w164 _ _ _ _ w216 w224 _ _ _ _ _ _ _ _ _ _ _ _ _ _ _ _ _ _ _ _ _ _ _ _ _ _]
      tunnel: w45 -> [_ _ _ _ _ w142 w162 _ _ _ _ _ _ _ _ w243 _ _ _ w273 w284 _ _ _ _ _ _ _ _ _ _ _ _ _ _ _ _ _ _]
      tunnel: w44 -> [_ _ _ _ _ w138 w159 _ _ _ _ _ _ _ _ _ w251 w258 w266 _ _ _ _ _ _ _ _ _ _ _ _ _ _ _ _ _ _ _ _]
      frame "Initialize" {
        w69 = UI_State."Idle"  # UI State
        # "Initialize - this message is sent when the message queue is created. Try to load the saved settings, and broadcast those settings to other loops."
        n22 = call "Load Settings from XML.vi"("Settings In"=w66) -> ("Settings Out"=w67:T8)  [unwired: 10 in]
        n23 = call "Enqueue Message (Array).vi"("error in (no error)"=w75, "Message Array"=string[] ["Init UI Refs"], "Message Queue"=w77) -> ("error out"=w74:errorcluster, "dup Message Queue"=w73:refnum<queue>)  [unwired: 7 in]
        n24 = call "Enqueue Message (Single).vi"("error in (no error)"=w74, "Message Data"="Ready..." ("Ready..."), "Message"="Update Status", "Message Queue"=w73) -> ("error out"=w70:errorcluster)  [unwired: 6 in, 1 out]
      }
      frame "Init UI Refs" {
        w102 = UI_State."Idle"  # UI State
        # "Init UI Refs - Store control references for UI controls.  Also enable/disable controls appropriately."
        n25 = control-ref of="Connect DMD"() -> (w80:refnum<vi>)
        n26 = control-ref of="Connect AOD"() -> (w78:refnum<vi>)
        n27 = control-ref of="Connect Camera"() -> (w93:refnum<vi>)
        n28 = control-ref of="Start"() -> (w100:refnum<vi>)
        n29 = control-ref of="DM Status"() -> (w86:refnum<vi>)
        n30 = control-ref of="Settings"() -> (w104:refnum<vi>)
        n31 = control-ref of="snap"() -> (w90:refnum<vi>)
        n32 = control-ref of="XYZ Status"() -> (w89:refnum<vi>)
        n33 = control-ref of="Status"() -> (w106:refnum<vi>)
        n34 = control-ref of="AOD Status"() -> (w79:refnum<vi>)
        n35 = control-ref of="Camera Status"() -> (w98:refnum<vi>)
        n36 = control-ref of="Stop"() -> (w105:refnum<vi>)
        n37 = control-ref of="V7001 Status"() -> (w81:refnum<vi>)
        n38 = control-ref of="Connect DM"() -> (w87:refnum<vi>)
        n39 = control-ref of="Exit"() -> (w103:refnum<vi>)
        n40 = control-ref of="Acquire frames"() -> (w92:refnum<vi>)
        n41 = control-ref of="Connect XYZ stage"() -> (w88:refnum<vi>)
        n42 = Bundle By Name(cluster=w101, "Camera Switch"=w93, "Camera Status Light Ref"=w98, "Start Ref"=w100, "Stop Ref"=w105, "Settings Ref"=w104, "Exit Ref"=w103, "Status Ref"=w106, "Acquire frames ref"=w92, "snap button ref"=w90, "XYZ Switch"=w88, "XYZ Status Light Ref"=w89, "DM Switch ref"=w87, "DM Status Light Ref"=w86, "V7001 Status Light Ref"=w81, "V7001 Switch Ref"=w80, "AOD Status Light Ref"=w79, "AOD Switch Ref"=w78) -> (w85:T15)
        n43 = control-ref of="Position in Microns"() -> (w82:refnum<vi>)
        n44 = control-ref of="Zernike Amplitudes"() -> (w83:refnum<vi>)
        n45 = Bundle By Name(cluster=w85, "Zernike Amplitudes"=w83, "Position in Microns"=w82) -> (w84:T15)
        n46 = call "UI Set State.vi"("error in (no error)"=w95, "State Type"=w94, "UI Refs"=w84) -> ("error out"=w96:errorcluster, "dup UI Refs"=w91:T15)  [unwired: 7 in]
        n47 = Merge Errors(w96) -> (w97:errorcluster)
      }
      frame "Update Status" {
        n48 = Variant To Data(error in=w111, type="", Variant=w112) -> (data=→"Status":string, error out=w110:errorcluster)
      }
      frame "Broadcast Settings" {
        w117 = "Update Settings" ("Message")
        # "Tell all the loops to deal with the new settings. Currently obsolte/unused"
        n49 = Unbundle By Name(w122) -> ("Camera Configuration"=w127:T9, "XYZ Configuration"=w125:T7, "DM Configuration"=w118:T11)
        n50 = call "Enqueue Message (Single).vi"("Message Data"=w118, "Message"=w117, "Message Queue"=w116) -> ("error out"=w115:errorcluster)  [unwired: 7 in, 1 out]
        n51 = call "Enqueue Message (Single).vi"("Message Data"=w125, "Message"=w117, "Message Queue"=w126) -> ("error out"=w119:errorcluster)  [unwired: 7 in, 1 out]
        n52 = call "Enqueue Message (Single).vi"("Message Data"=w127, "Message"=w117, "Message Queue"=w128) -> ("error out"=w120:errorcluster)  [unwired: 7 in, 1 out]
        n53 = Merge Errors(w120, w119, w115, w123) -> (w124:errorcluster)
      }
      frame "Error" {
        # "Error - Display an error dialog. This message is sent by the \"Error Handler\" VIs at the end of other loops in this application."
        n54 = Variant To Data(error in=w134, type=errorcluster {"status"=FALSE, "code"=0, "source"=""} ("error constant"), Variant=w133) -> (data=w135:errorcluster, error out=w132:errorcluster)
        n55 = call <vilib>:"Simple Error Handler.vi"("error in (no error)"=w135) -> ()  [unwired: 4 in, 5 out]
      }
      frame "Stop" {
        w139 = "Stop" ("Message")
        n56 = call "Enqueue Message (Single).vi"("error in (no error)"=w150, "Message"=w139, "Message Queue"=w151) -> ("error out"=w149:errorcluster)  [unwired: 7 in, 1 out]
        n57 = call "Enqueue Message (Single).vi"("error in (no error)"=w149, "Message"=w139, "Message Queue"=w148) -> ("error out"=w147:errorcluster)  [unwired: 7 in, 1 out]
        n58 = call "Enqueue Message (Single).vi"("error in (no error)"=w147, "Message"=w139, "Message Queue"=w146) -> ("error out"=w145:errorcluster)  [unwired: 7 in, 1 out]
        n59 = call "Enqueue Message (Single).vi"("error in (no error)"=w145, "Message"=w139, "Message Queue"=w144) -> ("error out"=w143:errorcluster)  [unwired: 7 in, 1 out]
        n60 = call "Enqueue Message (Single).vi"("error in (no error)"=w143, "Message"=w139, "Message Queue"=w142) -> ("error out"=w141:errorcluster)  [unwired: 7 in, 1 out]
        n61 = call "Enqueue Message (Single).vi"("error in (no error)"=w141, "Message"=w139, "Message Queue"=w138) -> ("error out"=w140:errorcluster)  [unwired: 7 in, 1 out]
        n62 = call "UI Set State.vi"("error in (no error)"=w140, "State Type"=w154, "UI Refs"=w153) -> ("error out"=w152:errorcluster)  [unwired: 7 in, 1 out]
      }
      frame "Exit" {
        w157 = TRUE ("Priority Message? (F)")
        w158 = "Exit" ("Message")
        w179 = UI_State."Idle"  # UI State
        # "Popup an error dialog if 'Exit' was called as a result of an error."
        # "Stop the VI"
        # "Exit - Send Exit messages to the Acquisition and Logging loops, and fire the user event to stop the Event Handling Loop."
        n63 = Variant To Data(type=errorcluster {"status"=FALSE, "code"=0, "source"=""} ("error constant"), Variant=w170) -> (data=w168:errorcluster)  [unwired: 1 in, 1 out]
        n64 = call <vilib>:"Simple Error Handler.vi"("error in (no error)"=w168) -> ()  [unwired: 4 in, 5 out]
        n65 = call "Enqueue Message (Single).vi"("Priority Message? (F)"=w157, "error in (no error)"=w176, "Message"=w158, "Message Queue"=w178) -> ("error out"=w175:errorcluster)  [unwired: 6 in, 1 out]
        n66 = call "Enqueue Message (Single).vi"("Priority Message? (F)"=w157, "error in (no error)"=w175, "Message"=w158, "Message Queue"=w177) -> ("error out"=w167:errorcluster)  [unwired: 6 in, 1 out]
        n67 = call "Enqueue Message (Single).vi"("Priority Message? (F)"=w157, "error in (no error)"=w167, "Message"=w158, "Message Queue"=w166) -> ("error out"=w165:errorcluster)  [unwired: 6 in, 1 out]
        n68 = call "Enqueue Message (Single).vi"("Priority Message? (F)"=w157, "error in (no error)"=w165, "Message"=w158, "Message Queue"=w164) -> ("error out"=w163:errorcluster)  [unwired: 6 in, 1 out]
        n69 = call "Enqueue Message (Single).vi"("Priority Message? (F)"=w157, "error in (no error)"=w163, "Message"=w158, "Message Queue"=w162) -> ("error out"=w161:errorcluster)  [unwired: 6 in, 1 out]
        n70 = call "Enqueue Message (Single).vi"("Priority Message? (F)"=w157, "error in (no error)"=w161, "Message"=w158, "Message Queue"=w159) -> ("error out"=w160:errorcluster)  [unwired: 6 in, 1 out]
        n71 = call "Fire User Event - Stop.vi"("error in (no error)"=w160, "User Event - Stop"=w174) -> ("error out"=w173:errorcluster)  [unwired: 9 in]
      }
      frame "Connect Camera" {
        n72 = call "Enqueue Message (Single).vi"("error in (no error)"=w183, "Message"="Connect", "Message Queue"=w185) -> ("error out"=w182:errorcluster)  [unwired: 7 in, 1 out]
      }
      frame "Start Live View" {
        n73 = call "Enqueue Message (Single).vi"("error in (no error)"=w191, "Message Data"=T3 {"Save?"=FALSE, "DCIMG Path"=path "", "Filename"="", "Total Frames"=0, "Sender"=enum."UI"} ("Acquisition Settings"), "Message"="Start Live View", "Message Queue"=w193) -> ("error out"=w190:errorcluster)  [unwired: 6 in, 1 out]
      }
      frame "Stop Live View" {
        n74 = call "Enqueue Message (Single).vi"("error in (no error)"=w198, "Message"="Stop Live View", "Message Queue"=w200) -> ("error out"=w197:errorcluster)  [unwired: 7 in, 1 out]
      }
      frame "Set Exposure" {
        n75 = call "Enqueue Message (Single).vi"("error in (no error)"=w206, "Message Data"=w204, "Message"="Set Exposure", "Message Queue"=w203) -> ("error out"=w205:errorcluster)  [unwired: 6 in, 1 out]
      }
      frame "Project Zernikes and record" {
        # "It is bad practice to have this automation code in the UI loop. Ultimately I will make an automation message loop, this is just from laziness"
        n76 = call "Enqueue Message (Single).vi"("error in (no error)"=w215, "Message Data"=w213, "Message"="Start Zernike Optimize", "Message Queue"=w216) -> ("error out"=w214:errorcluster)  [unwired: 6 in, 1 out]
      }
      frame "Take Z Stack" {
        # "It is bad practice to have this automation code in the UI loop. Ultimately I will make an automation message loop, this is just from laziness"
        n77 = call "Enqueue Message (Single).vi"("error in (no error)"=w223, "Message Data"=w221, "Message"="Start Z Stack", "Message Queue"=w224) -> ("error out"=w222:errorcluster)  [unwired: 6 in, 1 out]
      }
      frame "Connect XYZStage" {
        # "Connect to the stage, send the settings from the front panel"
        n78 = call "Enqueue Message (Single).vi"("error in (no error)"=w231, "Message Data"="XYZ Stage Configuration", "Message"="Connect", "Message Queue"=w228) -> ("error out"=w230:errorcluster)  [unwired: 6 in, 1 out]
      }
      frame "Connect DM" {
        # "Connect to the stage, send the settings from the front panel"
        n79 = call "Enqueue Message (Single).vi"("error in (no error)"=w239, "Message Data"="DM Serial", "Message"="Connect", "Message Queue"=w236) -> ("error out"=w238:errorcluster)  [unwired: 6 in, 1 out]
      }
      frame "Connect V7001" {
        # "Connect to the stage, send the settings from the front panel"
        n80 = call "Enqueue Message (Single).vi"("error in (no error)"=w246, "Message"="Connect", "Message Queue"=w243) -> ("error out"=w245:errorcluster)  [unwired: 7 in, 1 out]
      }
      frame "Connect AOD" {
        # "Connect to the stage, send the settings from the front panel"
        n81 = call "Enqueue Message (Single).vi"("error in (no error)"=w254, "Message Data"=w250, "Message"="Connect", "Message Queue"=w251) -> ("error out"=w253:errorcluster)  [unwired: 6 in, 1 out]
      }
      frame "Disconnect AOD" {
        # "Connect to the stage, send the settings from the front panel"
        n82 = call "Enqueue Message (Single).vi"("error in (no error)"=w261, "Message"="Stop", "Message Queue"=w258) -> ("error out"=w260:errorcluster)  [unwired: 7 in, 1 out]
      }
      frame "AOD XY" {
        # "Connect to the stage, send the settings from the front panel"
        n83 = call "Enqueue Message (Single).vi"("error in (no error)"=w269, "Message Data"=w265, "Message"="Set XY", "Message Queue"=w266) -> ("error out"=w268:errorcluster)  [unwired: 6 in, 1 out]
      }
      frame "Disconnect V7001" {
        # "Connect to the stage, send the settings from the front panel"
        n84 = call "Enqueue Message (Single).vi"("error in (no error)"=w276, "Message"="Stop", "Message Queue"=w273) -> ("error out"=w275:errorcluster)  [unwired: 7 in, 1 out]
      }
      frame "V7001 Test Frame" {
        n85 = call "Enqueue Message (Single).vi"("error in (no error)"=w282, "Message Data"=w280, "Message"="Test Frame", "Message Queue"=w284) -> ("error out"=w281:errorcluster)  [unwired: 6 in, 1 out]
      }
      frame "Disconnect DM" {
        # "Connect to the stage, send the settings from the front panel"
        n86 = call "Enqueue Message (Single).vi"("error in (no error)"=w291, "Message"="Stop", "Message Queue"=w288) -> ("error out"=w290:errorcluster)  [unwired: 7 in, 1 out]
      }
      frame "DM Zernike" {
        # "Connect to the stage, send the settings from the front panel"
        n87 = call "Enqueue Message (Single).vi"("error in (no error)"=w299, "Message Data"=w295, "Message"="Zernike", "Message Queue"=w296) -> ("error out"=w298:errorcluster)  [unwired: 6 in, 1 out]
      }
      frame "Set to current pos" {
        n88 = Variant To Data(error in=w304, type=refnum<vi> refnum ("XYZ start"), Variant=w311) -> (data=w310:refnum<vi>, error out=w305:errorcluster)
        n89 = Unbundle By Name(w308) -> ("Position in Microns"=w307:refnum<vi>)
        n90 = property class="Arr (strict)"(reference=w307, error in=w305) -> ("Value"=w306:dbl[])  [unwired: 2 out]
        n91 = property class="Arr (strict)"(reference=w310, "Value"=w306) -> (error out=w303:errorcluster)  [unwired: 1 in, 1 out]
      }
      frame "Zoom Sliders" {
        w324 = refnum<vi> refnum  # Slide
        n92 = Variant To Data(error in=w326, type=FALSE ("zoom sliders"), Variant=w330) -> (data=w318:bool, error out=w327:errorcluster)
        n93 = Unbundle By Name(w329) -> ("Zernike Amplitudes"=w328:refnum<vi>)
        n94 = case shown="True" w318 {
          tunnel: [1.0 ("y") 0.1 ("y")] -> w319
          frame False {
          }
          frame True {
          }
        }
        n95 = property class="Arr (strict)"(reference=w328, error in=w327) -> (error out=w317:errorcluster, "Array Element"=w323:refnum<vi>)  [unwired: 1 out]
        n96 = To More Specific Class(target class=w324, reference=w323, error in=w317) -> (specific class reference=w320:refnum<vi>, error out=w316:errorcluster)
        n97 = Multiply(x=w319, y=-1.0) -> (x*y=w321:dbl)
        n98 = property class="Slide"(reference=w320, error in=w316, "Scale.Minimum"=w321) -> (error out=w315:errorcluster)  [unwired: 1 out]
        n99 = property class="Slide"(reference=w320, error in=w315, "Scale.Maximum"=w319) -> (error out=w314:errorcluster)  [unwired: 1 out]
      }
      frame "Z from Paste" {
        # "This loop changes the zernike amplitudes, which  triggers an event to update the zernike modes"
        n100 = Variant To Data(error in=w343, type="" ("Message"), Variant=w344) -> (data=w338:string, error out=w342:errorcluster)
        n101 = Unbundle By Name(w346) -> ("Zernike Amplitudes"=w336:refnum<vi>)
        n102 = property class="Arr (strict)"(reference=w336) -> ("Value"=w335:dbl[])  [unwired: 1 in, 2 out]
        n103 = Spreadsheet String To Array(delimiter (Tab)="\n", format string="%e", spreadsheet string=w338, array type (2D Dbl)=w335) -> (array=w337:dbl[])
        n104 = property class="Arr (strict)"(reference=w336, error in=w342, "Val(Sgnl)"=w337) -> (error out=w345:errorcluster)  [unwired: 1 out]
      }
      frame "Disconnect XYZStage" {
        n105 = call "Enqueue Message (Single).vi"("error in (no error)"=w352, "Message"="Stop", "Message Queue"=w349) -> ("error out"=w351:errorcluster)  [unwired: 7 in, 1 out]
      }
      frame "poll position" {
        n106 = call "Enqueue Message (Single).vi"("error in (no error)"=w359, "Message"="Poll Position", "Message Queue"=w356) -> ("error out"=w358:errorcluster)  [unwired: 7 in, 1 out]
      }
      frame "Move To" {
        # "Tell XYZ Stage to move to new position"
        n107 = call "Enqueue Message (Single).vi"("error in (no error)"=w367, "Message Data"=w363, "Message"="Move To", "Message Queue"=w364) -> ("error out"=w366:errorcluster)  [unwired: 6 in, 1 out]
      }
      frame "Disconnect Camera" {
        n108 = call "Enqueue Message (Single).vi"("error in (no error)"=w373, "Message"="Disconnect", "Message Queue"=w375) -> ("error out"=w372:errorcluster)  [unwired: 7 in, 1 out]
      }
      frame "Acquire Frames" {
        # "Prepare camera to accept software triggers"
        n109 = call "Enqueue Message (Single).vi"("error in (no error)"=w381, "Message Data"=w378, "Message"="Acquire Frames", "Message Queue"=w383) -> ("error out"=w380:errorcluster)  [unwired: 6 in, 1 out]
      }
      frame "Snap" {
        # "Prepare camera to accept software triggers"
        n110 = call "Enqueue Message (Single).vi"("error in (no error)"=w389, "Message Data"=w386, "Message"="Snap", "Message Queue"=w391) -> ("error out"=w388:errorcluster)  [unwired: 6 in, 1 out]
      }
      frame "Camera Status" {
        n111 = Variant To Data(type=T17 {"Camera State"=enum."Idle", "Current Frame"=0, "Handle out"=0, "Camera Details"={"Model"="", "Camera ID"="", "Firmware"=""}, "Sub Region"={"H Offset"={"Value"=0, "Limits"={"Minimum"=0.0, "Maximum"=0.0, "Increment"=0.0}}, "V Offset"={"Value"=0, "Limits"={"Minimum"=0.0, "Maximum"=0.0, "Increment"=0.0}}, "H Size"={"Value"=0, "Limits"={"Minimum"=0.0, "Maximum"=0.0, "Increment"=0.0}}, "V Size"={"Value"=0, "Limits"={"Minimum"=0.0, "Maximum"=0.0, "Increment"=0.0}}}, "Acquisition Settings"={"Save?"=FALSE, "DCIMG Path"=path "", "Filename"="", "Total Frames"=0, "Sender"=enum."UI"}, "Live View State"={"Loop Counter"=0, "Time Of Latest Frame"=0, "Frame Count"=0, "FPS frames"=0.0, "FPS Time"=0, "Current FPS"=0.0}} ("Cluster"), Variant=w400) -> (data=w394:T17)  [unwired: 1 in, 1 out]
        n112 = Unbundle By Name(w394) -> ("Camera State"=w395:T18)
        n113 = case shown="\"Ready\"" w395 {
          tunnel: ["Connected" ("Camera Status") w416 "Disconnected" ("Camera Status")] -> w399
          tunnel: w398 -> [w409 w415 w422]
          tunnel: w394 -> [_ w419 _]
          frame "Ready" {
            n114 = Unbundle By Name(w409) -> ("Camera Status Light Ref"=w408:refnum<vi>, "Acquire frames ref"=w406:refnum<vi>, "snap button ref"=w404:refnum<vi>)
            n115 = property class="Bool"(reference=w408, "Value"=TRUE ("Enable?")) -> ()  [unwired: 1 in, 2 out]
            n116 = property class="Bool"(reference=w406, "DisabledEnum"=T21."Enabled" ("Disabled")) -> ()  [unwired: 1 in, 2 out]
            n117 = property class="Bool"(reference=w404, "DisabledEnum"=T21."Disabled and Grayed Out" ("Disabled")) -> ()  [unwired: 1 in, 2 out]
          }
          frame "Acquiring" {
            n118 = Unbundle By Name(w419) -> ("Acquisition Settings.Total Frames"=w417:i32, "Current Frame"=w418:i32)
            n119 = Unbundle By Name(w415) -> ("Acquire frames ref"=w414:refnum<vi>, "snap button ref"=w412:refnum<vi>)
            n120 = call "Build Text"("current"=w418, "total"=w417) -> ("Result"=w416:string)  [unwired: 12 in, 1 out]
            n121 = property class="Bool"(reference=w414, "DisabledEnum"=T21."Disabled and Grayed Out" ("Disabled")) -> ()  [unwired: 1 in, 2 out]
            n122 = property class="Bool"(reference=w412, "DisabledEnum"=T21."Enabled" ("Disabled")) -> ()  [unwired: 1 in, 2 out]
          }
          frame "Idle", Default {
            n123 = Unbundle By Name(w422) -> ("Camera Status Light Ref"=w424:refnum<vi>, "snap button ref"=w420:refnum<vi>)
            n124 = property class="Bool"(reference=w424, "Value"=FALSE ("Enable?")) -> ()  [unwired: 1 in, 2 out]
            n125 = property class="Bool"(reference=w420, "DisabledEnum"=T21."Disabled and Grayed Out" ("Disabled")) -> ()  [unwired: 1 in, 2 out]
          }
        }
        "Camera Status 3" <- w399
      }
      frame "DM Status" {
        # "To Do: fix the refs to the DM buttons, lights..."
        n126 = Variant To Data(type=T22 {"DM State"=enum."Idle", "Last Image Sent"=[], "Flatmap"=[], "Flatmap Path"=path "X:/Lab/Equipment/Boston Micromachines Multi-DM/Flash-Drive Contents/C187W147#040_Flat_Map/18W147#040_CLOSED_LOOP_VOLTAGES.txt", "Matlab Directory Path"=path "X:/Lab/Equipment/Boston Micromachines Multi-DM/Flash-Drive Contents/C187W147#040_Flat_Map/18W147#040_CLOSED_LOOP_VOLTAGES.txt"} ("Cluster"), Variant=w433) -> (data=w428:T22)  [unwired: 1 in, 1 out]
        n127 = Unbundle By Name(w428) -> ("DM State"=w429:T23, "Last Image Sent"=w426:dbl[][])
        n128 = case shown="\"Connected\"" w429 {
          tunnel: ["Connected" ("Camera Status") "Disconnected" ("Camera Status")] -> w432
          tunnel: w431 -> [w439 w441]
          tunnel: w428 -> [_ _]
          tunnel: w426 -> [w436 _]
          frame "Connected" {
            n129 = Unbundle By Name(w439) -> ("DM Status Light Ref"=w438:refnum<vi>)
            n130 = property class="Bool"(reference=w438, "Value"=TRUE ("Enable?")) -> ()  [unwired: 1 in, 2 out]
            "Intensity Graph" <- w436
          }
          frame "Idle", Default {
            n131 = Unbundle By Name(w441) -> ("DM Status Light Ref"=w443:refnum<vi>)
            n132 = property class="Bool"(reference=w443, "Value"=FALSE ("Enable?")) -> ()  [unwired: 1 in, 2 out]
          }
        }
        "DM Status" <- w432
      }
      frame "V7001 Status" {
        # "To Do: fix the refs to the DM buttons, lights..."
        n133 = Variant To Data(type=T24 {"V7001 State"=enum."Idle", "Handle out"=0, "Size"=[]} ("Cluster"), Variant=w451) -> (data=w446:T24)  [unwired: 1 in, 1 out]
        n134 = Unbundle By Name(w446) -> ("V7001 State"=w447:T25)
        n135 = case shown="\"Idle\", Default" w447 {
          tunnel: ["Connected" ("Camera Status") "Disconnected" ("Camera Status")] -> w450
          tunnel: w449 -> [w456 w458]
          tunnel: w446 -> [_ _]
          frame "Connected" {
            n136 = Unbundle By Name(w456) -> ("V7001 Status Light Ref"=w455:refnum<vi>)
            n137 = property class="Bool"(reference=w455, "Value"=TRUE ("Enable?")) -> ()  [unwired: 1 in, 2 out]
          }
          frame "Idle", Default {
            n138 = Unbundle By Name(w458) -> ("V7001 Status Light Ref"=w460:refnum<vi>)
            n139 = property class="Bool"(reference=w460, "Value"=FALSE ("Enable?")) -> ()  [unwired: 1 in, 2 out]
          }
        }
        "V7001 Status" <- w450
      }
      frame "AOD Status" {
        # "To Do: fix the refs to the DM buttons, lights..."
        n140 = Variant To Data(type=T26 {"AOD State"=enum."Idle", "daq task"="", "AOD Configuration"={"Physical Channel"="Dev1/ao0:1", "Maximum Value"=10.0, "Minimum Value"=1.0, "Update Rate"=192000.0}} ("Cluster"), Variant=w468) -> (data=w463:T26)  [unwired: 1 in, 1 out]
        n141 = Unbundle By Name(w463) -> ("AOD State"=w464:T27)
        n142 = case shown="\"Idle\", Default" w464 {
          tunnel: ["Connected" ("Camera Status") "Disconnected" ("Camera Status")] -> w467
          tunnel: w466 -> [w473 w475]
          tunnel: w463 -> [_ _]
          frame "Connected" {
            n143 = Unbundle By Name(w473) -> ("AOD Status Light Ref"=w472:refnum<vi>)
            n144 = property class="Bool"(reference=w472, "Value"=TRUE ("Enable?")) -> ()  [unwired: 1 in, 2 out]
          }
          frame "Idle", Default {
            n145 = Unbundle By Name(w475) -> ("AOD Status Light Ref"=w477:refnum<vi>)
            n146 = property class="Bool"(reference=w477, "Value"=FALSE ("Enable?")) -> ()  [unwired: 1 in, 2 out]
          }
        }
        "AOD Status" <- w467
      }
      frame "XYZStage Status" {
        n147 = Variant To Data(type=T28 {"XYZStage State"=enum."Idle", "Handle out"=0, "VISA resource name"="", "num controllers connected"=0, "Connector statuses"=[], "Position in Microns"=[], "measured manipulator"=0} ("Cluster"), Variant=w485) -> (data=w480:T28)  [unwired: 1 in, 1 out]
        n148 = Unbundle By Name(w480) -> ("XYZStage State"=w481:T29)
        n149 = case shown="\"Connected\"" w481 {
          tunnel: ["Connected" ("Camera Status") "" ("Camera Status") "Disconnected" ("Camera Status")] -> w484
          tunnel: w483 -> [w492 _ w495]
          tunnel: w480 -> [w489 _ _]
          frame "Connected" {
            # "Currently it sets button properties\neach time position is updated...\nchange this!"
            n150 = Unbundle By Name(w489) -> ("Position in Microns"=→"Position in Microns":dbl[])
            n151 = Unbundle By Name(w492) -> ("XYZ Status Light Ref"=w491:refnum<vi>)
            n152 = property class="Bool"(reference=w491, "Value"=TRUE ("Enable?")) -> ()  [unwired: 1 in, 2 out]
          }
          frame "Moving" {
          }
          frame "Idle", Default {
            n153 = Unbundle By Name(w495) -> ("XYZ Status Light Ref"=w497:refnum<vi>)  [unwired: 1 out]
            n154 = property class="Bool"(reference=w497, "Value"=FALSE ("Enable?")) -> ()  [unwired: 1 in, 2 out]
          }
        }
        "XYZ Status" <- w484
      }
      frame "Automation Status" {
        n155 = Variant To Data(type="" ("Message"), Variant=w503) -> (data=→"Automation Status":string)  [unwired: 1 in, 1 out]
      }
      frame Default {
        # "'Default' case only runs if there is a message that isn't defined in any of the other cases.  Output a programming error."
        n156 = xnode "Error Ring"("parameter 0"=w508) -> ("error out"=w507:errorcluster)
      }
    }
    n157 = call "Error Handler - Message Handling Loop.vi"("error in (no error)"=w62, "Message Queue"=w60) -> ("dup error in"=w61:errorcluster)  [unwired: 8 in, 1 out]
  }
  n158 = while {
    shift-right: [w523] -> w34
    shift-left: w35 -> [w524]
    tunnel: w6 -> [w521]
    tunnel: [w519] -> w32
    stop <- w522 stop-if-true
    # "Event Handling Loop"
    n159 = event shown="[15] \"Connect DM\": Value Change" {
      selector: w524 -> [_ _ _ _ _ _ _ _ _ _ _ _ _ _ _ _ _ _ _ _ _ _ _ _ _]
      dyn-events: [_ _ _ _ _ _ _ _ _ _ _ _ _ _ _ _ _ _ _ _ _ _ _ _ _] -> w523
      timeout: _ -> [_ _ _ _ _ _ _ _ _ _ _ _ _ _ _ _ _ _ _ _ _ _ _ _ _]
      tunnel: [_ _ _ _ _ _ _ _ _ _ _ _ _ _ _ _ _ _ _ _ _ _ _ _ TRUE] -> w522
      tunnel: [w525 w530 w535 w540 w544 w549 w554 w559 w564 _ _ _ w586 w603 w620 w637 w654 w672 w691 w707 w716 _ _ w738 w745] -> w520
      tunnel: w521 -> [w528 w531 w536 w541 w545 w550 w555 w560 w563 w570 w574 w578 w585 w602 w619 w636 w653 w671 w690 w709 w718 _ _ w740 w745]
      tunnel: [w526 w529 w534 w539 w543 w548 w553 w558 w565 w568 w573 w577 w582 w599 w616 w633 w650 w668 w688 w705 w714 _ w728 w736 _] -> w518
      event "Start": Value Change {
        n160 = event-data() -> ()  [unwired: 1 in, 1 out]
        n161 = call "Enqueue Message (Single).vi"("Message"="Start", "Message Queue"=w528) -> ("error out"=w526:errorcluster, "dup Message Queue"=w525:refnum<queue>)  [unwired: 8 in]
      }
      event "Stop": Value Change {
        n162 = event-data() -> ()  [unwired: 1 in, 1 out]
        n163 = call "Enqueue Message (Single).vi"("Message"="Stop", "Message Queue"=w531) -> ("error out"=w529:errorcluster, "dup Message Queue"=w530:refnum<queue>)  [unwired: 8 in]
      }
      event "zoom sliders": Value Change {
        n164 = event-data() -> ()  [unwired: 1 in, 2 out]
        n165 = call "Enqueue Message (Single).vi"("Message Data"="zoom sliders", "Message"="Zoom Sliders", "Message Queue"=w536) -> ("error out"=w534:errorcluster, "dup Message Queue"=w535:refnum<queue>)  [unwired: 7 in]
      }
      event "Acquire frames": Value Change {
        n166 = event-data() -> ()  [unwired: 1 in, 1 out]
        n167 = call "Enqueue Message (Single).vi"("Message Data"="Acquisition Settings", "Message"="Acquire Frames", "Message Queue"=w541) -> ("error out"=w539:errorcluster, "dup Message Queue"=w540:refnum<queue>)  [unwired: 7 in]
      }
      event "snap": Value Change {
        n168 = event-data() -> ()  [unwired: 1 in, 1 out]
        n169 = call "Enqueue Message (Single).vi"("Message"="Snap", "Message Queue"=w545) -> ("error out"=w543:errorcluster, "dup Message Queue"=w544:refnum<queue>)  [unwired: 8 in]
      }
      event "Move To": Value Change {
        n170 = event-data() -> ()  [unwired: 1 in, 1 out]
        n171 = call "Enqueue Message (Single).vi"("Message Data"="Position in Microns 2", "Message"="Move To", "Message Queue"=w550) -> ("error out"=w548:errorcluster, "dup Message Queue"=w549:refnum<queue>)  [unwired: 7 in]
      }
      event "Project and record": Value Change {
        n172 = event-data() -> ()  [unwired: 1 in, 1 out]
        n173 = call "Enqueue Message (Single).vi"("Message Data"="ZO Settings", "Message"="Project Zernikes and record", "Message Queue"=w555) -> ("error out"=w553:errorcluster, "dup Message Queue"=w554:refnum<queue>)  [unwired: 7 in]
      }
      event "Exposure": Value Change {
        n174 = event-data() -> ()  [unwired: 1 in, 2 out]
        n175 = call "Enqueue Message (Single).vi"("Message Data"="Exposure", "Message"="Set Exposure", "Message Queue"=w560) -> ("error out"=w558:errorcluster, "dup Message Queue"=w559:refnum<queue>)  [unwired: 7 in]
      }
      event "Exit": Value Change {
        # "The UI Message Loop handles sending the Exit message to other loops."
        n176 = event-data() -> ()  [unwired: 1 in, 1 out]
        n177 = call "Enqueue Message (Single).vi"("Priority Message? (F)"=TRUE, "Message Data"=errorcluster {"status"=FALSE, "code"=0, "source"=""} ("error constant"), "Message"="Exit", "Message Queue"=w563) -> ("error out"=w565:errorcluster, "dup Message Queue"=w564:refnum<queue>)  [unwired: 6 in]
      }
      event "Start at Current Pos": Value Change {
        # "This event is sending a reference to the array that is to be modified"
        n178 = event-data() -> ()  [unwired: 1 in, 2 out]
        n179 = control-ref of="XYZ start"() -> (w569:refnum<vi>)
        n180 = call "Enqueue Message (Single).vi"("Message Data"=w569, "Message"="Set to current pos", "Message Queue"=w570) -> ("error out"=w568:errorcluster)  [unwired: 7 in, 1 out]
      }
      event "Stop at Current Pos": Value Change {
        # "This event is sending a reference to the array that is to be modified"
        n181 = event-data() -> ()  [unwired: 1 in, 2 out]
        n182 = control-ref of="XYZ end"() -> (w572:refnum<vi>)
        n183 = call "Enqueue Message (Single).vi"("Message Data"=w572, "Message"="Set to current pos", "Message Queue"=w574) -> ("error out"=w573:errorcluster)  [unwired: 7 in, 1 out]
      }
      event "Take Z Stack": Value Change {
        n184 = event-data() -> ()  [unwired: 1 in, 2 out]
        n185 = call "Enqueue Message (Single).vi"("Message Data"="Zstack Settings", "Message"="Take Z Stack", "Message Queue"=w578) -> ("error out"=w577:errorcluster)  [unwired: 7 in, 1 out]
      }
      event "Connect Camera": Value Change {
        # "The UI Message Loop handles sending the Exit message to other loops."
        n186 = event-data() -> ("CtlRef"=w584:refnum<vi>)  [unwired: 1 in]
        n187 = case shown="False" "Connect Camera" {
          tunnel: [w590 w595] -> w581
          tunnel: [w589 w594] -> w586
          tunnel: w585 -> [w588 w593]
          tunnel: [TRUE ("Value") FALSE ("Value")] -> w583
          frame True {
            n188 = call "Enqueue Message (Single).vi"("Message"="Connect Camera", "Message Queue"=w588) -> ("error out"=w590:errorcluster, "dup Message Queue"=w589:refnum<queue>)  [unwired: 8 in]
          }
          frame False {
            n189 = call "Enqueue Message (Single).vi"("Message"="Disconnect Camera", "Message Queue"=w593) -> ("error out"=w595:errorcluster, "dup Message Queue"=w594:refnum<queue>)  [unwired: 8 in]
          }
        }
        n190 = property class="Bool (strict)"(reference=w584, error in=w581, "Value"=w583) -> (error out=w582:errorcluster)  [unwired: 1 out]
      }
      event "Go Live": Value Change {
        # "The UI Message Loop handles sending the Exit message to other loops."
        n191 = event-data() -> ("CtlRef"=w601:refnum<vi>)  [unwired: 1 in]
        n192 = case shown="True" "Go Live" {
          tunnel: [w607 w612] -> w598
          tunnel: [w606 w611] -> w603
          tunnel: w602 -> [w605 w610]
          tunnel: [TRUE ("Value") FALSE ("Value")] -> w600
          frame True {
            n193 = call "Enqueue Message (Single).vi"("Message"="Start Live View", "Message Queue"=w605) -> ("error out"=w607:errorcluster, "dup Message Queue"=w606:refnum<queue>)  [unwired: 8 in]
          }
          frame False {
            n194 = call "Enqueue Message (Single).vi"("Message"="Stop Live View", "Message Queue"=w610) -> ("error out"=w612:errorcluster, "dup Message Queue"=w611:refnum<queue>)  [unwired: 8 in]
          }
        }
        n195 = property class="Bool (strict)"(reference=w601, error in=w598, "Value"=w600) -> (error out=w599:errorcluster)  [unwired: 1 out]
      }
      event "Connect XYZ stage": Value Change {
        n196 = event-data() -> ("CtlRef"=w618:refnum<vi>)  [unwired: 1 in]
        n197 = case shown="False" "Connect XYZ stage" {
          tunnel: [w624 w629] -> w615
          tunnel: [w623 w628] -> w620
          tunnel: w619 -> [w622 w627]
          tunnel: [TRUE ("Value") FALSE ("Value")] -> w617
          frame True {
            n198 = call "Enqueue Message (Single).vi"("Message"="Connect XYZStage", "Message Queue"=w622) -> ("error out"=w624:errorcluster, "dup Message Queue"=w623:refnum<queue>)  [unwired: 8 in]
          }
          frame False {
            n199 = call "Enqueue Message (Single).vi"("Message"="Disconnect XYZStage", "Message Queue"=w627) -> ("error out"=w629:errorcluster, "dup Message Queue"=w628:refnum<queue>)  [unwired: 8 in]
          }
        }
        n200 = property class="Bool (strict)"(reference=w618, error in=w615, "Value"=w617) -> (error out=w616:errorcluster)  [unwired: 1 out]
      }
      event "Connect DM": Value Change {
        n201 = event-data() -> ("CtlRef"=w635:refnum<vi>)  [unwired: 1 in]
        n202 = case shown="True" "Connect DM" {
          tunnel: [w641 w646] -> w632
          tunnel: [w640 w645] -> w637
          tunnel: w636 -> [w639 w644]
          tunnel: [TRUE ("Value") FALSE ("Value")] -> w634
          frame True {
            n203 = call "Enqueue Message (Single).vi"("Message"="Connect DM", "Message Queue"=w639) -> ("error out"=w641:errorcluster, "dup Message Queue"=w640:refnum<queue>)  [unwired: 8 in]
          }
          frame False {
            n204 = call "Enqueue Message (Single).vi"("Message"="Disconnect DM", "Message Queue"=w644) -> ("error out"=w646:errorcluster, "dup Message Queue"=w645:refnum<queue>)  [unwired: 8 in]
          }
        }
        n205 = property class="Bool (strict)"(reference=w635, error in=w632, "Value"=w634) -> (error out=w633:errorcluster)  [unwired: 1 out]
      }
      event "Connect DMD": Value Change {
        n206 = event-data() -> ("CtlRef"=w652:refnum<vi>)  [unwired: 1 in]
        n207 = case shown="False" "Connect DMD" {
          tunnel: [w658 w663] -> w649
          tunnel: [w657 w662] -> w654
          tunnel: w653 -> [w656 w661]
          tunnel: [TRUE ("Value") FALSE ("Value")] -> w651
          frame True {
            n208 = call "Enqueue Message (Single).vi"("Message"="Connect V7001", "Message Queue"=w656) -> ("error out"=w658:errorcluster, "dup Message Queue"=w657:refnum<queue>)  [unwired: 8 in]
          }
          frame False {
            n209 = call "Enqueue Message (Single).vi"("Message"="Disconnect V7001", "Message Queue"=w661) -> ("error out"=w663:errorcluster, "dup Message Queue"=w662:refnum<queue>)  [unwired: 8 in]
          }
        }
        n210 = property class="Bool (strict)"(reference=w652, error in=w649, "Value"=w651) -> (error out=w650:errorcluster)  [unwired: 1 out]
      }
      event "Connect AOD": Value Change {
        n211 = event-data() -> ("CtlRef"=w670:refnum<vi>)  [unwired: 1 in]
        n212 = case shown="True" "Connect AOD" {
          tunnel: [w677 w682] -> w667
          tunnel: [w676 w681] -> w672
          tunnel: w671 -> [w675 w680]
          tunnel: [TRUE ("Value") FALSE ("Value")] -> w669
          tunnel: "AOD Configuration" -> [w673 _]
          frame True {
            n213 = call "Enqueue Message (Single).vi"("Message Data"=w673, "Message"="Connect AOD", "Message Queue"=w675) -> ("error out"=w677:errorcluster, "dup Message Queue"=w676:refnum<queue>)  [unwired: 7 in]
          }
          frame False {
            n214 = call "Enqueue Message (Single).vi"("Message"="Disconnect AOD", "Message Queue"=w680) -> ("error out"=w682:errorcluster, "dup Message Queue"=w681:refnum<queue>)  [unwired: 8 in]
          }
        }
        n215 = property class="Bool (strict)"(reference=w670, error in=w667, "Value"=w669) -> (error out=w668:errorcluster)  [unwired: 1 out]
      }
      event "Test Frame", "Frame": Value Change {
        n216 = event-data() -> ()  [unwired: 1 in, 2 out]
        n217 = control-ref of="Test Frame"() -> (w684:refnum<vi>)
        n218 = case shown="True" "Test Frame" {
          tunnel: [w697 w702] -> w687
          tunnel: [w696 w701] -> w691
          tunnel: w690 -> [w695 w700]
          tunnel: [TRUE ("Value") FALSE ("Value")] -> w689
          tunnel: "Frame" -> [w692 _]
          frame True {
            n219 = call "Enqueue Message (Single).vi"("Message Data"=w692, "Message"="V7001 Test Frame", "Message Queue"=w695) -> ("error out"=w697:errorcluster, "dup Message Queue"=w696:refnum<queue>)  [unwired: 7 in]
          }
          frame False {
            w698 = u16 0 items=["All Off", "All On", "Checkerboard 1", "Random"] ("Frame")
            n220 = call "Enqueue Message (Single).vi"("Message Data"=w698, "Message"="V7001 Test Frame", "Message Queue"=w700) -> ("error out"=w702:errorcluster, "dup Message Queue"=w701:refnum<queue>)  [unwired: 7 in]
          }
        }
        n221 = property class="Bool (strict)"(reference=w684, error in=w687, "Value"=w689) -> (error out=w688:errorcluster)  [unwired: 1 out]
      }
      event "Zernike Amplitudes": Value Change {
        n222 = event-data() -> ()  [unwired: 1 in, 1 out]
        n223 = call "Enqueue Message (Single).vi"("Message Data"="Zernike Amplitudes", "Message"="DM Zernike", "Message Queue"=w709) -> ("error out"=w706:errorcluster, "dup Message Queue"=w707:refnum<queue>)  [unwired: 7 in]
        n224 = case shown="No Error" w706 {
          selector: w706 -> [w711 w712]
          tunnel: [w711 w712] -> w705
          frame No Error {
            n225 = Wait (ms)(milliseconds to wait=u32 100) -> ()  [unwired: 1 out]
          }
          frame Error {
          }
        }
      }
      event "X,Y": Value Change {
        (unwired) dbl[] [-0.010101010101010055, 0.0010101010101010027, 0.0, 0.0, 0.0, -0.06565656565656566, 0.0, 0.0, 0.043434343434343436, 0.0, 0.0, 0.0, 0.0, 0.0, 0.0] ("X,Y")
        n226 = event-data() -> ()  [unwired: 1 in, 1 out]
        n227 = call "Enqueue Message (Single).vi"("Message Data"="X,Y", "Message"="AOD XY", "Message Queue"=w718) -> ("error out"=w715:errorcluster, "dup Message Queue"=w716:refnum<queue>)  [unwired: 7 in]
        n228 = case shown="No Error" w715 {
          selector: w715 -> [w720 w721]
          tunnel: [w720 w721] -> w714
          frame No Error {
            n229 = Wait (ms)(milliseconds to wait=u32 100) -> ()  [unwired: 1 out]
          }
          frame Error {
          }
        }
      }
      event "Zero zernike": Value Change {
        n230 = event-data() -> ()  [unwired: 1 in, 2 out]
        n231 = control-ref of="Zernike Amplitudes"() -> (w723:refnum<vi>)
        n232 = property class="Arr (strict)"(reference=w723, "Val(Sgnl)"=dbl[] [0.0, 0.0, 0.0, 0.0, 0.0, 0.0, 0.0, 0.0, 0.0, 0.0, 0.0, 0.0, 0.0, 0.0, 0.0] ("Zernike Amplitudes 2")) -> ()  [unwired: 1 in, 2 out]
      }
      event "Sliders to text": Value Change {
        n233 = event-data() -> ()  [unwired: 1 in, 2 out]
        n234 = control-ref of="Zernike Amplitudes"() -> (w734:refnum<vi>)
        n235 = property class="Arr (strict)"(reference=w734) -> (error out=w729:errorcluster, "Value"=w733:dbl[])  [unwired: 1 in, 1 out]
        n236 = Array To Spreadsheet String(delimiter (Tab)="\n", array=w733, 3:"%2.5f" ("format string")) -> (spreadsheet string=w727:string)
        n237 = control-ref of="Matlab Paste"() -> (w730:refnum<vi>)
        n238 = String Length(string=w727) -> (length=w726:i32)
        n239 = Decrement(x=w726) -> (x-1=w725:i32)
        n240 = String Subset(string=w727, length (rest)=w725) -> (substring=w724:string)  [unwired: 1 in]
        n241 = property class="Str"(reference=w730, error in=w729, "Value"=w724) -> (error out=w728:errorcluster)  [unwired: 1 out]
      }
      event "Set Z from paste": Value Change {
        n242 = event-data() -> ()  [unwired: 1 in, 2 out]
        n243 = call "Enqueue Message (Single).vi"("Message Data"="Matlab Paste", "Message"="Z from Paste", "Message Queue"=w740) -> ("error out"=w737:errorcluster, "dup Message Queue"=w738:refnum<queue>)  [unwired: 7 in]
        n244 = case shown="No Error" w737 {
          selector: w737 -> [w742 w743]
          tunnel: [w742 w743] -> w736
          frame No Error {
            n245 = Wait (ms)(milliseconds to wait=u32 100) -> ()  [unwired: 1 out]
          }
          frame Error {
          }
        }
      }
      event User Event {
        # "The Message Handling Loop processed an \"Exit\" message, which fired this event to stop the Event Handling Loop."
        n246 = event-data() -> ()  [unwired: 1 in, 1 out]
        n247 = local write "Status"("Exit" ("Exit String")) -> ()
      }
    }
    n248 = call "Error Handler - Event Handling Loop.vi"("error in (no error)"=w518, "Message Queue"=w520) -> ("dup error in"=w519:errorcluster)  [unwired: 8 in, 1 out]
  }
  n249 = Unregister For Events(event registration refnum=w34, error in=w32) -> (error out=w31:errorcluster)
  n250 = Release Queue(queue=w6, error in (no error)=w29) -> (error out=w16:errorcluster)  [unwired: 1 in, 2 out]
  n251 = Release Notifier(notifier=w13, error in (no error)=w16) -> (error out=w10:errorcluster)  [unwired: 1 in, 2 out]
  n252 = Release Notifier(notifier=w8, error in (no error)=w10) -> (error out=w9:errorcluster)  [unwired: 1 in, 2 out]
  n253 = Merge Errors(w31, w9, w22, w21, w20, w15, w7, w2) -> (w30:errorcluster)
  n254 = call "Destroy User Event - Stop.vi"("error in (no error)"=w30, "User Event - Stop"=w24) -> ()  [unwired: 9 in, 1 out]
